vi "Result inspection.vi"(7 "입력 클러스터":T1, 8 "error in":errorcluster caption="에러 입력(에러 없음)", 9 "Ref. Data (excluded)":refnum<vi>[](array[refnum]), 10 "Ref. Data (Inspection)":refnum<vi>[](array[refnum]), 11 "Func ext":string) -> (0 "error out":errorcluster caption="에러 출력", 1 "Data 3D":string[][][][](array[string]), 2 "Data (spec 미적용)":string[][](array[string]), 3 "Data (spec 적용)":string[][](array[string]))   [LabVIEW 2020]
uses:
  Controls/Clst_Result inspec.ctl
  Controls/Cmd_Var Data IO.ctl
  Variables/Global_Cal Info.vi
  Public/Polymorph/Rmv Empt Arr_2D Str.vi
  Public/Polymorph/Cell Space_Table.vi
  Public/Polymorph/Data Class_2D Str.vi
  <vilib>/express/express arith-compare/Formula/XNode/ExpressFormulaBlockNode.xnode
panel:
  out "spec DBL":dbl[][][](array[numeric])
  out "Spec":string[][](array[string])
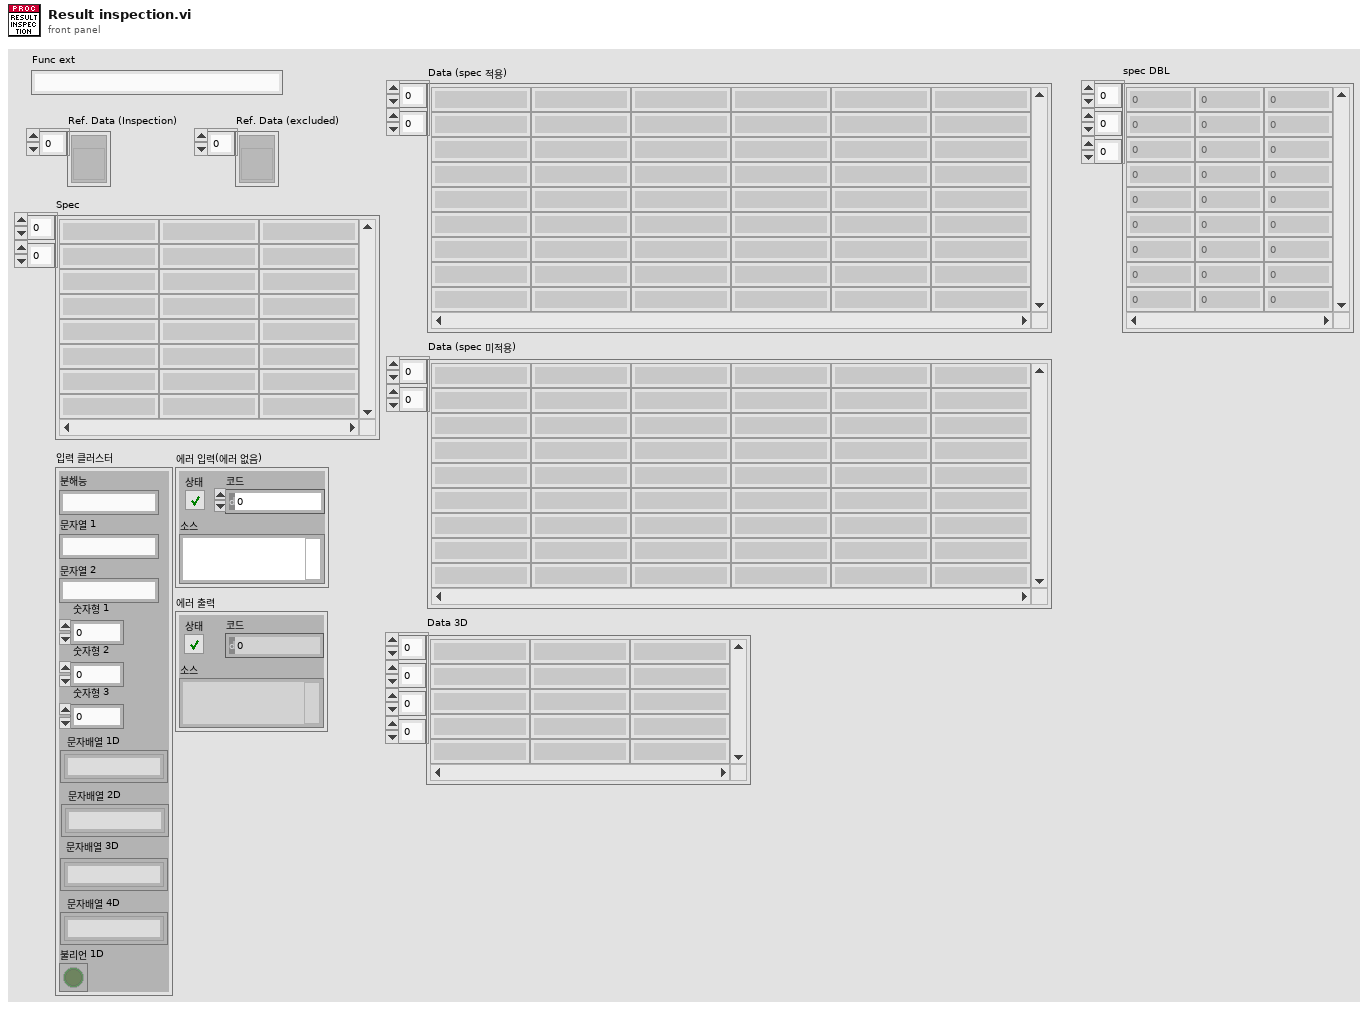
[diagram p1: front panel]
types:
  T1 = typedef "Clst_Result inspec.ctl" = cluster{"분해능":string, "문자열 1":string, "문자열 2":string, "숫자형 1":i32, "숫자형 2":i32, "숫자형 3":dbl, "문자배열 1D":string[], "문자배열 2D":string[][], "문자배열 3D":string[][][], "문자배열 4D":string[][][][], "불리언 1D":bool[]}
  T2 = typedef "Cmd_Var Data IO.ctl" = enum16{"Condition", "Condition Default", "Condition_Temp", "Resolution", "Resolution Default", "Resolution Old", "Spec", "Spec Default", "Spec Old", "Spec Temp", "Result", "Result2", "Result3", "Result_Temp", "Result_ADJ", "Result_ADJ2", "STD1", "STD2", "STD3", "STD4", "STD5", "STD Temp", "CMC", "CMC Default"}
  T3 = cluster{"세부분류코드":string, "형식":string, "옵션":string, "측정기명":string, "EXCEL파일명":string, "TEMP":string}
  T4 = enum8{"Enabled", "Disabled", "Disabled and Grayed Out"}
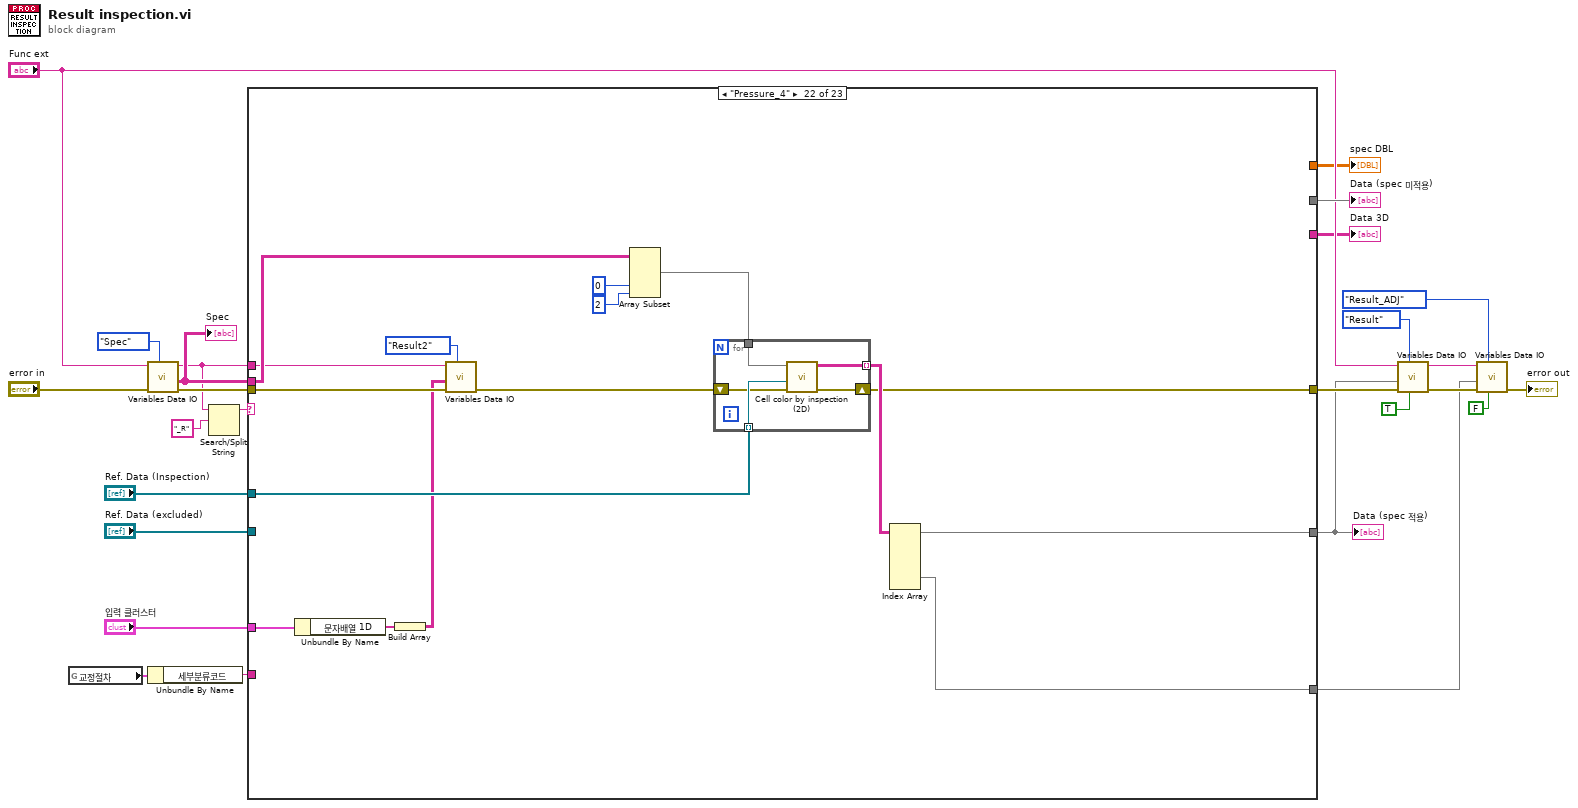
[diagram p0: block diagram]
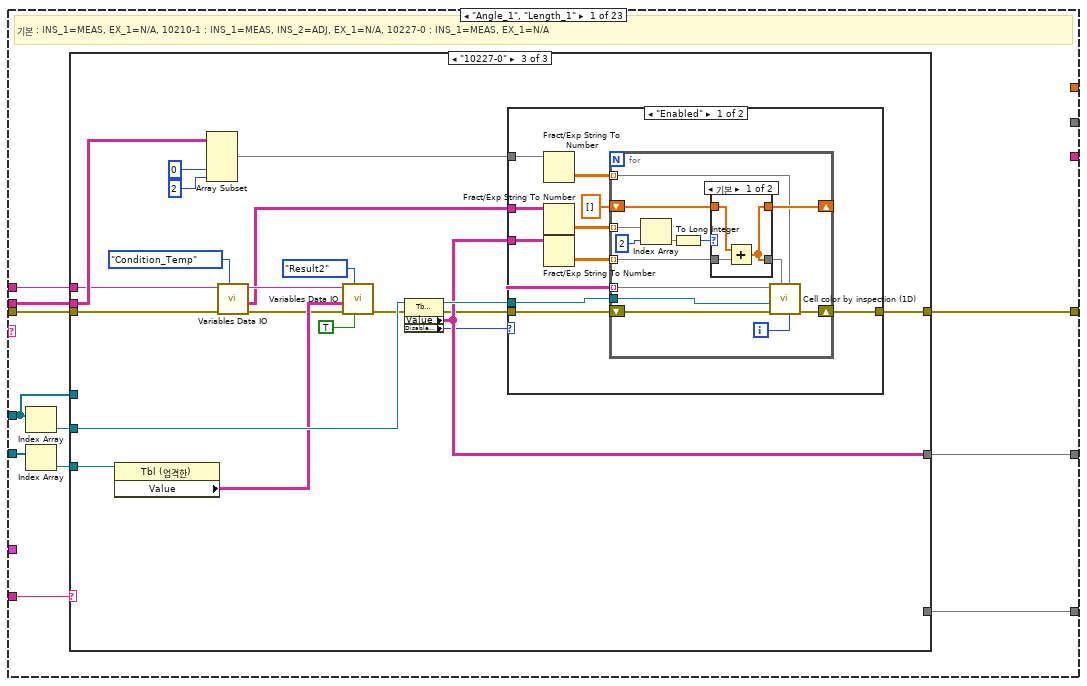
[diagram p2: hidden frame]
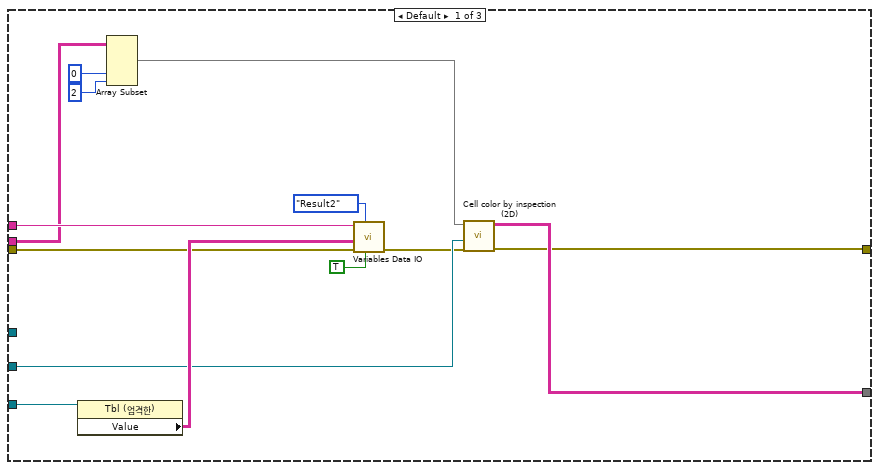
[diagram p3: hidden frame]
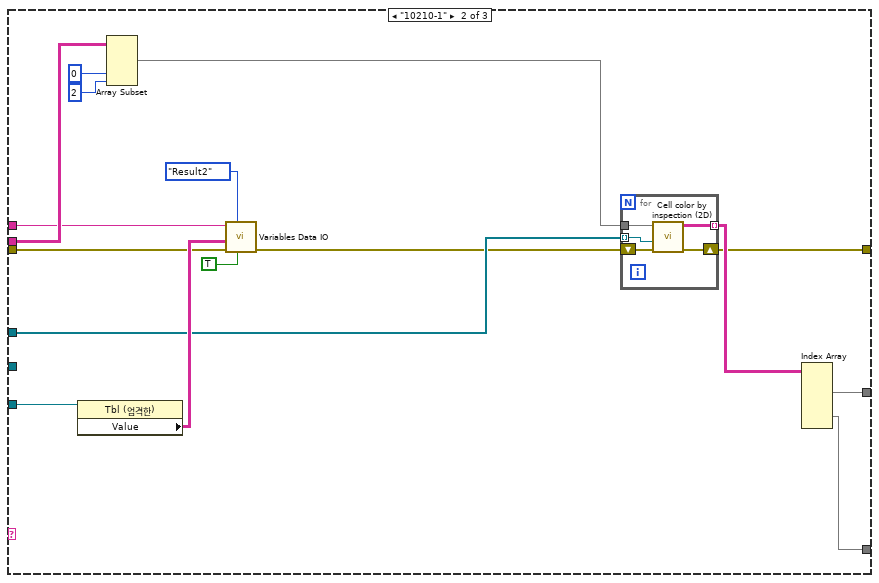
[diagram p4: hidden frame]
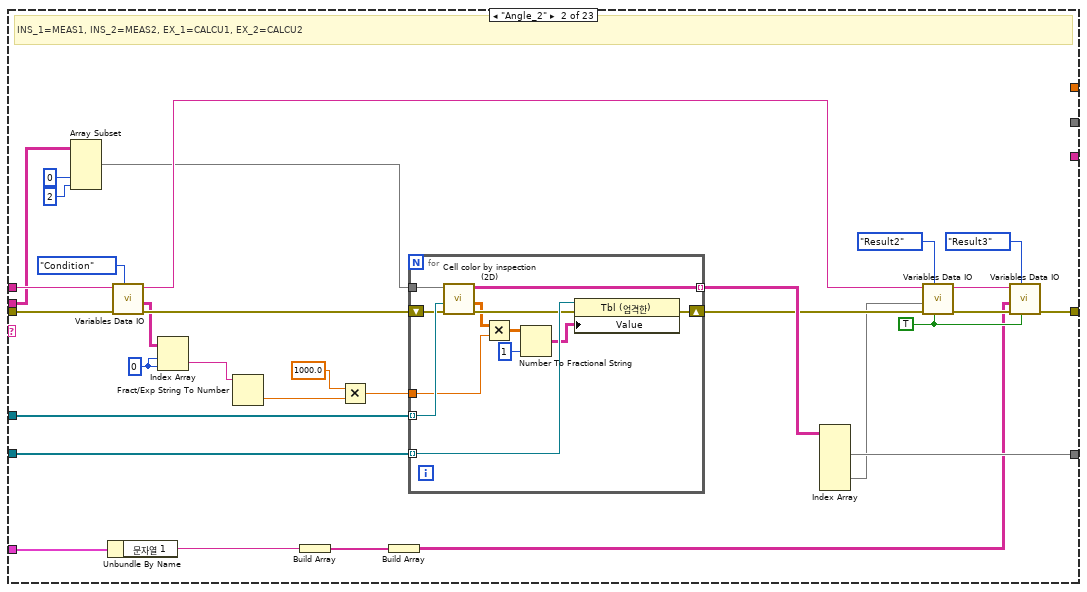
[diagram p7: hidden frame]
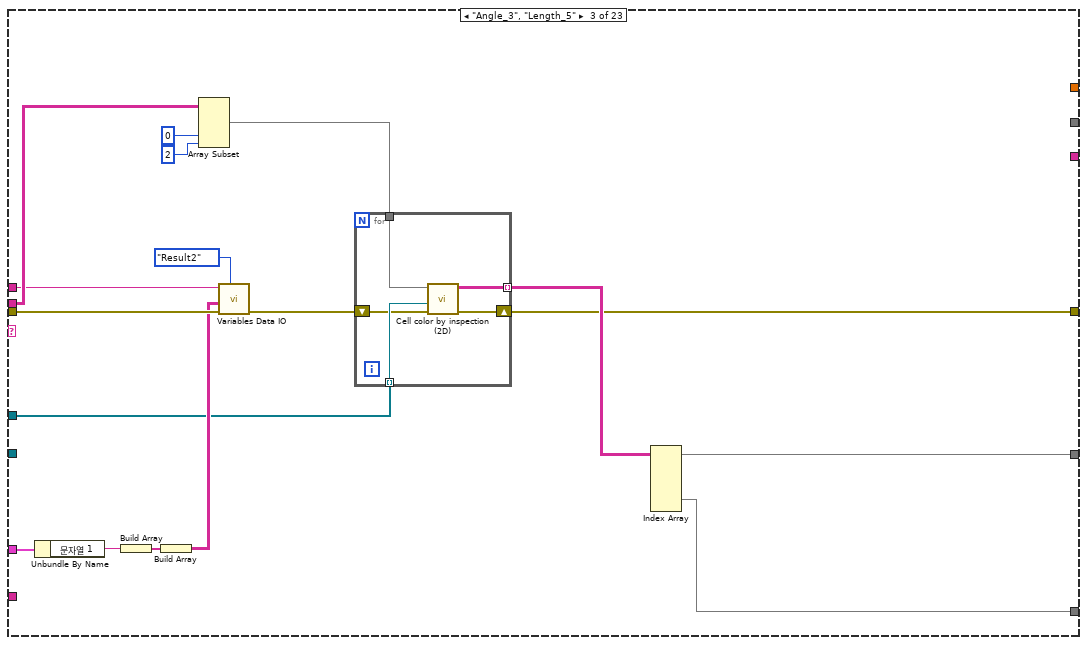
[diagram p8: hidden frame]
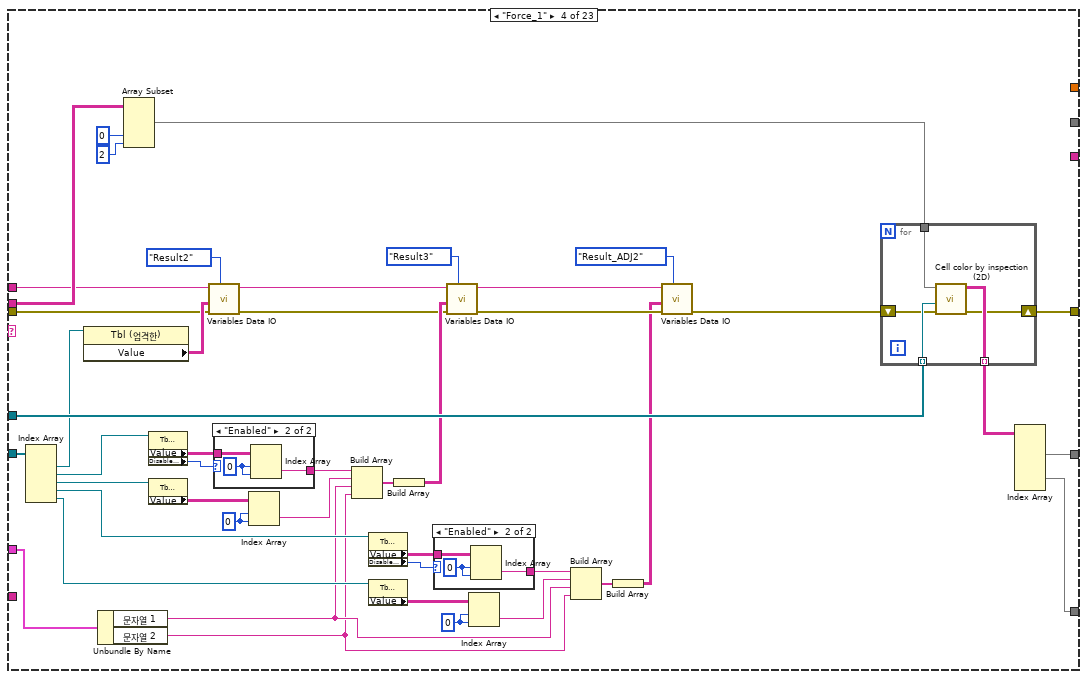
[diagram p9: hidden frame]
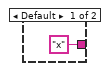
[diagram p10: hidden frame]
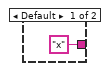
[diagram p11: hidden frame]
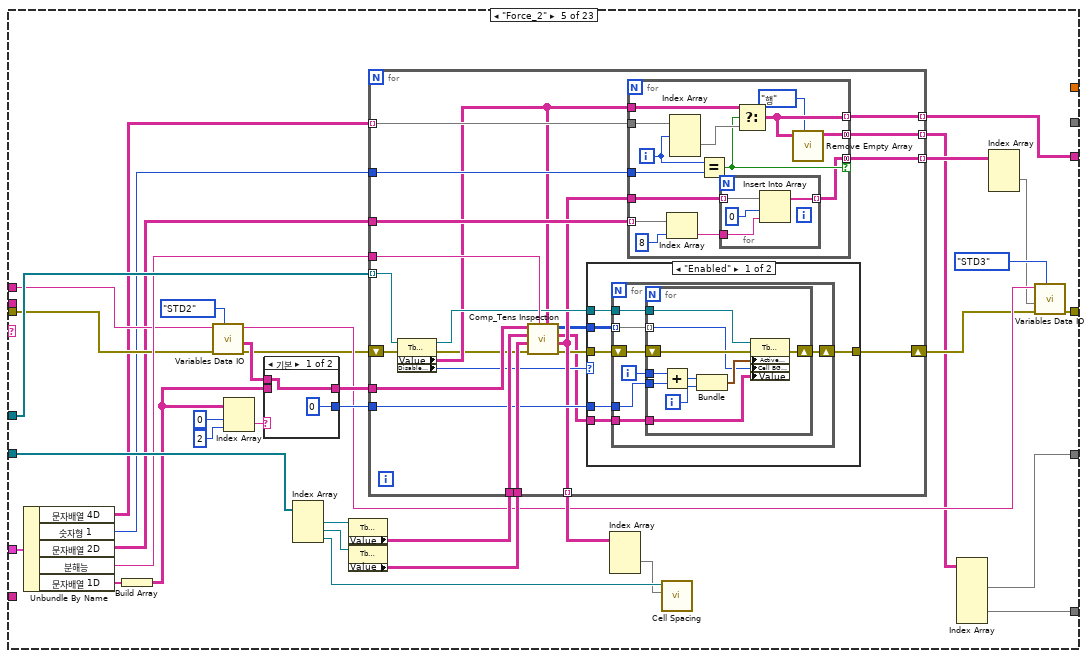
[diagram p12: hidden frame]
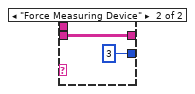
[diagram p14: hidden frame]
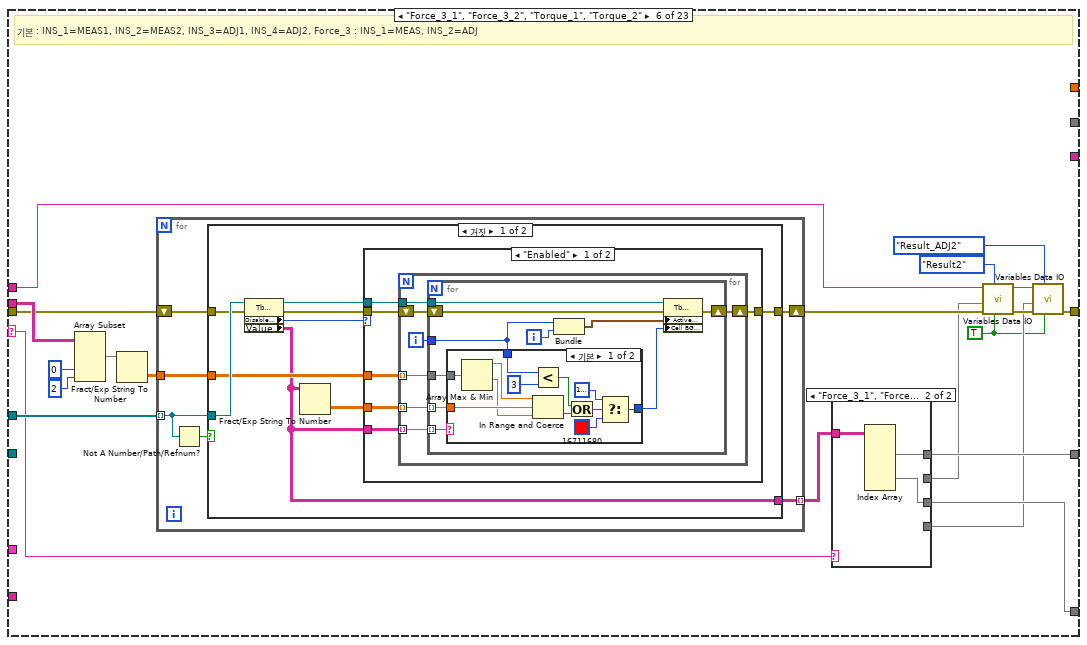
[diagram p15: hidden frame]
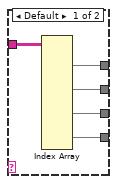
[diagram p16: hidden frame]
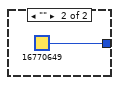
[diagram p17: hidden frame]
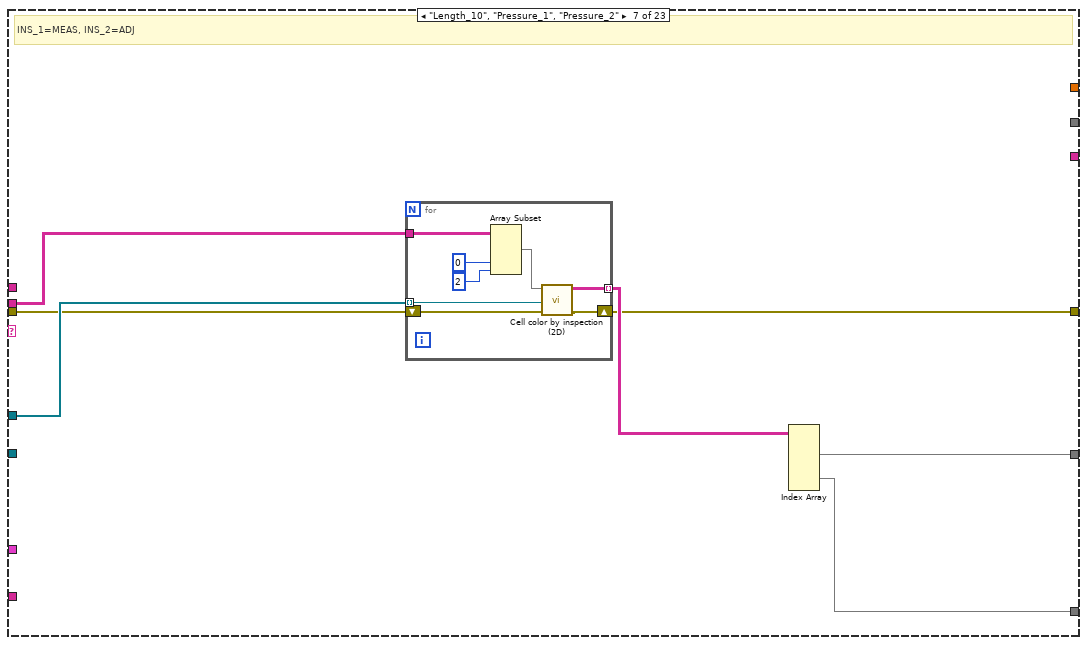
[diagram p20: hidden frame]
diagram:
  n1 = global read "Global_Cal Info.vi" "교정절차"() -> (w10:T3)
  n2 = call "Variables Data IO.vi"("Select"=Cmd_Var_Data_IO."Spec", "error in"="error in", "Func_ext"="Func ext") -> ("error out"=w19:errorcluster, "Data Out"=w17:string[][], "Func_ext Out"=w11:string)  [unwired: 6 in]
  "Spec" <- w17
  n3 = Unbundle By Name(w10) -> ("세부분류코드"=w9:string)
  n4 = Search/Split String(string=w11, search string/char (-)="_R" ("검색 문자열/문자 (-)")) -> (substring before match=w12:string)  [unwired: 1 in, 2 out]
  n5 = case shown="\"Pressure_4\"" w12 {
    selector: w12 -> [_ _ _ _ _ w350 _ _ _ _ _ _ _ _ _ _ _ _ _ _ _ _ _]
    tunnel: w19 -> [w31 w146 w175 w211 w273 w363 w436 w481 w559 w584 w641 w1221 w1258 w1298 w1353 w1411 w1441 w1461 w1514 w1585 w1673 w1691 w1719]
    tunnel: [w30 w131 w168 w206 w253 w356 w433 w448 w536 w579 w622 w1222 w1256 w1294 w1337 w1408 w1443 w1458 w1534 w1615 w1667 w1695 w1709] -> w24
    tunnel: "Ref. Data (Inspection)" -> [w28 w153 w171 w232 w281 w364 w438 w480 w560 w580 w649 w1243 w1260 w1313 w1356 w1415 w1444 w1454 w1542 w1623 w1670 w1697 w1721]
    tunnel: "Ref. Data (excluded)" -> [w34 w147 _ w227 w279 _ _ w483 w551 w577 w648 w1229 w1270 _ w1355 w1410 w1442 w1489 w1505 w1612 _ _ _]
    tunnel: [w36 w151 w167 w205 w247 w360 w434 w475 w534 w578 w610 w1223 w1262 w1310 w1359 w1414 w1439 w1456 w1532 w1613 w1666 w1694 w1717] -> w21
    tunnel: [_ _ _ _ _ _ _ _ _ _ w612 _ _ _ _ _ _ _ w1527 w1606 _ _ _] -> w20
    tunnel: w17 -> [w35 w140 w180 w229 _ w366 w437 w484 w544 w581 w650 w1240 w1265 w1306 w1358 w1413 _ w1469 w1540 w1621 w1678 w1699 w1720]
    tunnel: "입력 클러스터" -> [_ w133 w179 w213 w278 _ _ _ w552 _ w637 w1233 w1272 w1302 _ _ _ w1475 w1516 w1582 w1677 w1692 _]
    tunnel: w11 -> [w32 w145 w177 w212 w272 w351 _ w477 w557 _ w638 w1220 w1276 w1297 w1354 w1409 _ w1462 w1515 w1584 w1675 w1690 w1714]
    tunnel: w9 -> [w29 _ _ _ _ _ _ _ _ _ _ _ _ _ _ w1397 _ _ _ _ _ _ _]
    tunnel: [w27 _ w166 w204 w246 w358 w432 w459 _ _ _ _ w1261 _ _ _ _ w1455 _ _ w1665 w1693 _] -> w4
    tunnel: [_ _ _ _ w257 _ _ _ _ _ _ _ _ _ _ _ _ _ _ _ _ _ _] -> w2
    tunnel: [_ _ _ _ _ _ _ _ _ w576 _ _ _ _ _ _ _ _ _ _ _ _ _] -> w1
    frame "Angle_1", "Length_1" {
      # "기본 : INS_1=MEAS, EX_1=N/A, 10210-1 : INS_1=MEAS, INS_2=ADJ, EX_1=N/A, 10227-0 : INS_1=MEAS, EX_1=N/A"
      n6 = Index Array(array=w28) -> (element=w37:refnum<vi>)  [unwired: 1 in]
      n7 = Index Array(array=w34) -> (element=w33:refnum<vi>)  [unwired: 1 in]
      n8 = case shown="\"10227-0\"" w29 {
        tunnel: w37 -> [w42 _ w93]
        tunnel: [w41 w56 w81] -> w36
        tunnel: w35 -> [w44 w65 w89]
        tunnel: w33 -> [w49 w63 w88]
        tunnel: w32 -> [w47 w61 w84]
        tunnel: w31 -> [w40 w54 w74]
        tunnel: [w38 w52 w78] -> w30
        tunnel: w28 -> [_ w58 _]
        tunnel: [_ w55 _] -> w27
        frame Default {
          n9 = property class="Tbl (엄격한)"(reference=w49) -> ("Value"=w45:string[][])  [unwired: 1 in, 2 out]
          n10 = Array Subset(array=w44, index (col)=0 ("인덱스"), length (col)=2 ("길이")) -> (w43:string[][])  [unwired: 2 in]
          n11 = call "Variables Data IO.vi"("Write blank data ?(F)"=TRUE ("Write blank data ?(T)"), "Select"=Cmd_Var_Data_IO."Result2", "error in"=w40, "Data In"=w45, "Func_ext"=w47) -> ("error out"=w39:errorcluster)  [unwired: 4 in, 2 out]
          n12 = call "Cell color by inspection (2D).vi"("에러 입력(에러 없음)"=w39, "테이블 입력"=w42, "Spec"=w43) -> ("에러 출력"=w38:errorcluster, "Data(str)"=w41:string[][])  [unwired: 6 in, 1 out]
        }
        frame "10210-1" {
          n13 = property class="Tbl (엄격한)"(reference=w63) -> ("Value"=w59:string[][])  [unwired: 1 in, 2 out]
          n14 = Array Subset(array=w65, index (col)=0 ("인덱스"), length (col)=2 ("길이")) -> (w64:string[][])  [unwired: 2 in]
          n15 = call "Variables Data IO.vi"("Write blank data ?(F)"=TRUE ("Write blank data ?(T)"), "Select"=Cmd_Var_Data_IO."Result2", "error in"=w54, "Data In"=w59, "Func_ext"=w61) -> ("error out"=w53:errorcluster)  [unwired: 4 in, 2 out]
          n16 = for {
            tunnel: [w69] -> w57 mode=indexing
            tunnel: w64 -> [w72]
            tunnel: w58 -> [w70] mode=indexing
            shift-right: [w68] -> w52
            shift-left: w53 -> [w71]
            n17 = call "Cell color by inspection (2D).vi"("에러 입력(에러 없음)"=w71, "테이블 입력"=w70, "Spec"=w72) -> ("에러 출력"=w68:errorcluster, "Data(str)"=w69:string[][])  [unwired: 6 in, 1 out]
          }
          n18 = Index Array(array=w57) -> (element #1=w56:string[][], element #2=w55:string[][])  [unwired: 6 in]
        }
        frame "10227-0" {
          n19 = property class="Tbl (엄격한)"(reference=w88) -> ("Value"=w85:string[][])  [unwired: 1 in, 2 out]
          n20 = Array Subset(array=w89, index (col)=0 ("인덱스"), length (col)=2 ("길이")) -> (w79:string[][])  [unwired: 2 in]
          n21 = call "Variables Data IO.vi"("Select"=Cmd_Var_Data_IO."Condition_Temp", "error in"=w74, "Func_ext"=w84) -> ("error out"=w75:errorcluster, "Data Out"=w80:string[][], "Func_ext Out"=w83:string)  [unwired: 6 in]
          n22 = call "Variables Data IO.vi"("Write blank data ?(F)"=TRUE ("Write blank data ?(T)"), "Select"=Cmd_Var_Data_IO."Result2", "error in"=w75, "Data In"=w85, "Func_ext"=w83) -> ("error out"=w76:errorcluster)  [unwired: 4 in, 2 out]
          n23 = property class="Tbl (엄격한)"(reference=w93, error in=w76) -> (reference out=w92:refnum<vi>, error out=w77:errorcluster, "Value"=w81:string[][], "DisabledEnum"=w73:T4)
          n24 = case shown="\"Enabled\"" w73 {
            tunnel: w92 -> [w102 _]
            tunnel: w81 -> [w101 _]
            tunnel: w80 -> [w100 _]
            tunnel: w79 -> [w99 _]
            tunnel: [w95 w123] -> w78
            tunnel: w77 -> [w94 w123]
            frame "Enabled" {
              n25 = Fract/Exp String To Number(string=w99) -> (number=w103:dbl[][])  [unwired: 3 in, 1 out]
              n26 = Fract/Exp String To Number(string=w100) -> (number=w96:dbl[][])  [unwired: 3 in, 1 out]
              n27 = Fract/Exp String To Number(string=w101) -> (number=w98:dbl[][])  [unwired: 3 in, 1 out]
              n28 = for {
                tunnel: w103 -> [w110] mode=indexing
                tunnel: w98 -> [w116] mode=indexing
                tunnel: w102 -> [w107]
                tunnel: w101 -> [w106] mode=indexing
                shift-right: [w105] -> w95
                shift-left: w94 -> [w108]
                shift-right: [w111] -> _
                shift-left: dbl[] [] -> [w117]
                tunnel: w96 -> [w113] mode=indexing
                i -> [w104]
                n29 = Index Array(array=w113, index=2 ("인덱스")) -> (element=w115:dbl)
                n30 = To Long Integer(number=w115) -> (32bit integer=w112:i32)
                n31 = case shown="기본" w112 {
                  tunnel: w116 -> [w119 w122]
                  tunnel: [w118 w122] -> w109
                  tunnel: w117 -> [w120 w121]
                  tunnel: [w118 w121] -> w111
                  frame Default {
                    n32 = Add(x=w120, y=w119) -> (x+y=w118:dbl[])
                  }
                  frame 0 {
                  }
                }
                n33 = call "Cell color by inspection (1D).vi"("행번호"=w104, "Spec"=w110, "Data (DBL)"=w109, "에러 입력"=w108, "테이블 입력"=w107, "Data (str)"=w106) -> ("에러 출력"=w105:errorcluster)  [unwired: 5 in]
              }
            }
            frame Default {
            }
          }
        }
      }
    }
    frame "Angle_2" {
      w138 = 0 ("인덱스 (열)")
      w130 = TRUE ("Write blank data ?")
      # "INS_1=MEAS1, INS_2=MEAS2, EX_1=CALCU1, EX_2=CALCU2"
      n34 = Array Subset(array=w140, index (col)=0 ("인덱스"), length (col)=2 ("길이")) -> (w124:string[][])  [unwired: 2 in]
      n35 = Unbundle By Name(w133) -> ("문자열 1"=w127:string)
      n36 = call "Variables Data IO.vi"("Select"=Cmd_Var_Data_IO."Condition", "error in"=w146, "Func_ext"=w145) -> ("Data Out"=w142:string[][], "Func_ext Out"=w144:string)  [unwired: 6 in, 1 out]
      n37 = Index Array(array=w142, index (row)=w138, index (col)=w138) -> (element=w137:string)
      n38 = Fract/Exp String To Number(string=w137) -> (number=w136:dbl)  [unwired: 3 in, 1 out]
      n39 = Build Array(w127) -> (w126:string[])
      n40 = Multiply(x=1000.0 ("y"), y=w136) -> (x*y=w135:dbl)
      n41 = Build Array(w126) -> (w125:string[][])
      n42 = for {
        tunnel: w153 -> [w165] mode=indexing
        tunnel: [w159] -> w152 mode=indexing
        shift-right: [w160] -> w149
        shift-left: w146 -> [w164]
        tunnel: w147 -> [w162] mode=indexing
        tunnel: w124 -> [w163]
        tunnel: w135 -> [w157]
        n43 = call "Cell color by inspection (2D).vi"("에러 입력(에러 없음)"=w164, "테이블 입력"=w165, "Spec"=w163) -> ("에러 출력"=w161:errorcluster, "Data(DBL)"=w158:dbl[][], "Data(str)"=w159:string[][])  [unwired: 6 in]
        n44 = Multiply(x=w158, y=w157) -> (x*y=w156:dbl[][])
        n45 = Number To Fractional String(number=w156, precision (6)=i16 1 ("정밀도(6)")) -> (F-format string=w154:string[][])  [unwired: 2 in]
        n46 = property class="Tbl (엄격한)"(reference=w162, error in=w161, "Value"=w154) -> (error out=w160:errorcluster)  [unwired: 1 out]
      }
      n47 = Index Array(array=w152) -> (element #1=w151:string[][], element #2=w148:string[][])  [unwired: 6 in]
      n48 = call "Variables Data IO.vi"("Write blank data ?(F)"=w130, "Select"=Cmd_Var_Data_IO."Result2", "error in"=w149, "Data In"=w148, "Func_ext"=w144) -> ("error out"=w132:errorcluster, "Func_ext Out"=w128:string)  [unwired: 4 in, 1 out]
      n49 = call "Variables Data IO.vi"("Write blank data ?(F)"=w130, "Select"=Cmd_Var_Data_IO."Result3", "error in"=w132, "Data In"=w125, "Func_ext"=w128) -> ("error out"=w131:errorcluster)  [unwired: 4 in, 2 out]
    }
    frame "Angle_3", "Length_5" {
      n50 = Unbundle By Name(w179) -> ("문자열 1"=w176:string)
      n51 = Build Array(w176) -> (w174:string[])
      n52 = Build Array(w174) -> (w173:string[][])
      n53 = Array Subset(array=w180, index (col)=0 ("인덱스"), length (col)=2 ("길이")) -> (w172:string[][])  [unwired: 2 in]
      n54 = call "Variables Data IO.vi"("Select"=Cmd_Var_Data_IO."Result2", "error in"=w175, "Data In"=w173, "Func_ext"=w177) -> ("error out"=w170:errorcluster)  [unwired: 5 in, 2 out]
      n55 = for {
        tunnel: w172 -> [w187]
        tunnel: w171 -> [w186] mode=indexing
        tunnel: [w184] -> w169 mode=indexing
        shift-right: [w183] -> w168
        shift-left: w170 -> [w185]
        n56 = call "Cell color by inspection (2D).vi"("에러 입력(에러 없음)"=w185, "테이블 입력"=w186, "Spec"=w187) -> ("에러 출력"=w183:errorcluster, "Data(str)"=w184:string[][])  [unwired: 6 in, 1 out]
      }
      n57 = Index Array(array=w169) -> (element #1=w167:string[][], element #2=w166:string[][])  [unwired: 6 in]
    }
    frame "Force_1" {
      w196 = 0 ("인덱스 (행)")
      w218 = 0 ("인덱스 (행)")
      n58 = Index Array(array=w227) -> (element #1=w226:refnum<vi>, element #2=w224:refnum<vi>, element #3=w223:refnum<vi>, element #4=w192:refnum<vi>, element #5=w191:refnum<vi>)  [unwired: 5 in]
      n59 = property class="Tbl (엄격한)"(reference=w226) -> ("Value"=w225:string[][])  [unwired: 1 in, 2 out]
      n60 = Unbundle By Name(w213) -> ("문자열 1"=w189:string, "문자열 2"=w188:string)
      n61 = Array Subset(array=w229, index (col)=0 ("인덱스"), length (col)=2 ("길이")) -> (w209:string[][])  [unwired: 2 in]
      n62 = property class="Tbl (엄격한)"(reference=w224) -> ("Value"=w220:string[][], "DisabledEnum"=w221:T4)  [unwired: 1 in, 2 out]
      n63 = property class="Tbl (엄격한)"(reference=w223) -> ("Value"=w217:string[][])  [unwired: 1 in, 2 out]
      n64 = call "Variables Data IO.vi"("Select"=Cmd_Var_Data_IO."Result2", "error in"=w211, "Data In"=w225, "Func_ext"=w212) -> ("error out"=w207:errorcluster, "Func_ext Out"=w210:string)  [unwired: 5 in, 1 out]
      n65 = case shown="\"Enabled\"" w221 {
        tunnel: w220 -> [_ w245]
        tunnel: ["ⅹ" w243] -> w219
        frame Default {
        }
        frame "Enabled" {
          w244 = 0 ("인덱스 (행)")
          n66 = Index Array(array=w245, index (row)=w244, index (col)=w244) -> (element=w243:string)
        }
      }
      n67 = Index Array(array=w217, index (row)=w218, index (col)=w218) -> (element=w216:string)
      n68 = Build Array(w219, w216, w189, w188) -> (w215:string[])
      n69 = property class="Tbl (엄격한)"(reference=w192) -> ("Value"=w194:string[][], "DisabledEnum"=w193:T4)  [unwired: 1 in, 2 out]
      n70 = property class="Tbl (엄격한)"(reference=w191) -> ("Value"=w197:string[][])  [unwired: 1 in, 2 out]
      n71 = Build Array(w215) -> (w214:string[][])
      n72 = case shown="\"Enabled\"" w193 {
        tunnel: w194 -> [_ w236]
        tunnel: ["ⅹ" w234] -> w195
        frame Default {
        }
        frame "Enabled" {
          w235 = 0 ("인덱스 (행)")
          n73 = Index Array(array=w236, index (row)=w235, index (col)=w235) -> (element=w234:string)
        }
      }
      n74 = call "Variables Data IO.vi"("Select"=Cmd_Var_Data_IO."Result3", "error in"=w207, "Data In"=w214, "Func_ext"=w210) -> ("error out"=w202:errorcluster, "Func_ext Out"=w200:string)  [unwired: 5 in, 1 out]
      n75 = Index Array(array=w197, index (row)=w196, index (col)=w196) -> (element=w198:string)
      n76 = Build Array(w195, w198, w189, w188) -> (w199:string[])
      n77 = Build Array(w199) -> (w190:string[][])
      n78 = call "Variables Data IO.vi"("Select"=Cmd_Var_Data_IO."Result_ADJ2", "error in"=w202, "Data In"=w190, "Func_ext"=w200) -> ("error out"=w201:errorcluster)  [unwired: 5 in, 2 out]
      n79 = for {
        tunnel: w209 -> [w241]
        tunnel: w232 -> [w240] mode=indexing
        tunnel: [w239] -> w208 mode=indexing
        shift-right: [w237] -> w206
        shift-left: w201 -> [w238]
        n80 = call "Cell color by inspection (2D).vi"("에러 입력(에러 없음)"=w238, "테이블 입력"=w240, "Spec"=w241) -> ("에러 출력"=w237:errorcluster, "Data(str)"=w239:string[][])  [unwired: 6 in, 1 out]
      }
      n81 = Index Array(array=w208) -> (element #1=w205:string[][], element #2=w204:string[][])  [unwired: 6 in]
    }
    frame "Force_2" {
      n82 = Unbundle By Name(w278) -> ("문자배열 4D"=w260:string[][][][], "숫자형 1"=w261:i32, "문자배열 2D"=w262:string[][], "분해능"=w274:string, "문자배열 1D"=w267:string[])
      n83 = Build Array(w267) -> (w263:string[][])
      n84 = call "Variables Data IO.vi"("Select"=Cmd_Var_Data_IO."STD2", "error in"=w273, "Func_ext"=w272) -> ("error out"=w252:errorcluster, "Data Out"=w265:string[][], "Func_ext Out"=w254:string)  [unwired: 6 in]
      n85 = Index Array(array=w263, index (row)=0 ("비활성화된 인덱스 (행)"), index (col)=2 ("비활성화된 인덱스 (열)")) -> (element=w268:string)
      n86 = case shown="기본" w268 {
        tunnel: w263 -> [_ w349]
        tunnel: [w347 w349] -> w266
        tunnel: w265 -> [w347 _]
        tunnel: [0 ("x") 3 ("x")] -> w264
        frame Default {
        }
        frame "Force Measuring Device" {
        }
      }
      n87 = Index Array(array=w279) -> (element #1=w280:refnum<vi>, element #2=w277:refnum<vi>, element #3=w259:refnum<vi>)  [unwired: 3 in]
      n88 = property class="Tbl (엄격한)"(reference=w280) -> ("Value"=w276:string[][])  [unwired: 1 in, 2 out]
      n89 = property class="Tbl (엄격한)"(reference=w277) -> ("Value"=w275:string[][])  [unwired: 1 in, 2 out]
      n90 = for {
        tunnel: w276 -> [w303]
        tunnel: w275 -> [w302]
        tunnel: w274 -> [w301]
        tunnel: w266 -> [w300]
        tunnel: w264 -> [w299]
        tunnel: w262 -> [w298]
        tunnel: w261 -> [w297]
        tunnel: w260 -> [w296] mode=indexing
        tunnel: [w293] -> w258 mode=indexing
        tunnel: [w292] -> w257 mode=indexing
        tunnel: w281 -> [w291] mode=indexing
        tunnel: [w290] -> w255 mode=indexing
        shift-right: [w287] -> w251
        shift-left: w252 -> [w289]
        tunnel: [w286] -> w248 mode=indexing
        n91 = property class="Tbl (엄격한)"(reference=w291, error in=w289) -> (reference out=w295:refnum<vi>, error out=w288:errorcluster, "Value"=w294:string[][], "DisabledEnum"=w285:T4)
        n92 = call "Comp_Tens Inspection.vi"("Value"=w294, "분해능"=w301, "error in (no error)"=w288, "Spec"=w302, "Condition"=w303, "STD"=w300) -> ("error out"=w283:errorcluster, "사용기준추"=w293:string[][], "Value out"=w282:string[][], "색상 배열"=w284:u32[][])  [unwired: 2 in]
        n93 = case shown="\"Enabled\"" w285 {
          tunnel: w299 -> [w309 _]
          tunnel: w295 -> [w308 _]
          tunnel: [w307 w327] -> w287
          tunnel: w284 -> [w306 _]
          tunnel: w283 -> [w305 w327]
          tunnel: w282 -> [w304 _]
          frame "Enabled" {
            n94 = for {
              tunnel: w306 -> [w316] mode=indexing
              tunnel: w308 -> [w315]
              shift-right: [w312] -> w307
              shift-left: w305 -> [w313]
              tunnel: w304 -> [w311]
              tunnel: w309 -> [w310]
              i -> [w314]
              n95 = for {
                tunnel: w316 -> [w319] mode=indexing
                tunnel: w315 -> [w326]
                tunnel: w314 -> [w321]
                shift-right: [w322] -> w312
                shift-left: w313 -> [w323]
                tunnel: w311 -> [w318]
                tunnel: w310 -> [w317]
                i -> [w325]
                n96 = Add(x=w321, y=w317) -> (x+y=w320:i32)
                n97 = Bundle(w320, w325) -> (w324:cluster{i32, i32})  [unwired: 1 in]
                n98 = property class="Tbl (엄격한)"(reference=w326, error in=w323, "Active Cell"=w324, "Cell BG Color"=w319, "Value"=w318) -> (error out=w322:errorcluster)  [unwired: 1 out]
              }
            }
          }
          frame Default {
          }
        }
        n99 = for {
          tunnel: w296 -> [w340]
          tunnel: w294 -> [w337]
          tunnel: w297 -> [w341]
          tunnel: [w336] -> w292 mode=indexing
          tunnel: w298 -> [w330] mode=indexing
          tunnel: [w335] -> w286 mode=concatenating
          tunnel: w293 -> [w332]
          tunnel: [w331] -> w290 mode=concatenating if=w333
          i -> [w339]
          n100 = Index Array(array=w330, index=8 ("비활성화된 인덱스 (열)")) -> (element=w328:string)
          n101 = Index Array(array=w340, index (dim 0)=w339) -> (element=w338:string[][])  [unwired: 2 in]
          n102 = Equal?(x=w339, y=w341) -> (x = y?=w333:bool)
          n103 = for {
            tunnel: w332 -> [w345] mode=indexing
            tunnel: w328 -> [w344]
            tunnel: [w342] -> w331 mode=indexing
            n104 = Insert Into Array(array=w345, index=0 ("인덱스"), new element=w344) -> (w342:string[])
          }
          n105 = Select(t=w337, s=w333, f=w338) -> (s? t:f=w336:string[][])
          n106 = call-poly "Remove Empty Array.vi"("조건"=enum16{"행", "열", "행,열"}."행", "Data in"=w336) -> ("Data out"=w335:string[][])  [unwired: 8 in, 1 out]
        }
      }
      n107 = Index Array(array=w258) -> (element=w249:string[][])  [unwired: 3 in]
      n108 = call-poly "Cell Spacing.vi"("Data in"=w249, "테이블 참조 in"=w259) -> ()  [unwired: 7 in, 3 out]
      n109 = Index Array(array=w248) -> (element #1=w247:string[][], element #2=w246:string[][])  [unwired: 6 in]
      n110 = Index Array(array=w255) -> (element=w250:string[][])  [unwired: 3 in]
      n111 = call "Variables Data IO.vi"("Select"=Cmd_Var_Data_IO."STD3", "error in"=w251, "Data In"=w250, "Func_ext"=w254) -> ("error out"=w253:errorcluster)  [unwired: 5 in, 2 out]
    }
    frame "Force_3_1", "Force_3_2", "Torque_1", "Torque_2" {
      w352 = TRUE ("Clear data ?")
      # "기본 : INS_1=MEAS1, INS_2=MEAS2, INS_3=ADJ1, INS_4=ADJ2, Force_3 : INS_1=MEAS, INS_2=ADJ"
      n112 = Array Subset(array=w366, index (col)=0 ("인덱스"), length (col)=2 ("길이")) -> (w369:string[][])  [unwired: 2 in]
      n113 = Fract/Exp String To Number(string=w369) -> (number=w365:dbl[][])  [unwired: 3 in, 1 out]
      n114 = for {
        tunnel: w364 -> [w384] mode=indexing
        tunnel: w365 -> [w382]
        tunnel: [w381] -> w361 mode=indexing
        shift-right: [w379] -> w362
        shift-left: w363 -> [w380]
        n115 = Not A Number/Path/Refnum?(number/path/refnum=w384) -> (NaN/Path/Refnum?=w383:bool)
        n116 = case shown="거짓" w383 {
          tunnel: w382 -> [w391 _]
          tunnel: [w390 _] -> w381
          tunnel: w384 -> [w393 _]
          tunnel: w380 -> [w388 w431]
          tunnel: [w386 w431] -> w379
          frame False {
            n117 = property class="Tbl (엄격한)"(reference=w393, error in=w388) -> (reference out=w392:refnum<vi>, error out=w387:errorcluster, "DisabledEnum"=w385:T4, "Value"=w390:string[][])
            n118 = Fract/Exp String To Number(string=w390) -> (number=w389:dbl[][])  [unwired: 3 in, 1 out]
            n119 = case shown="\"Enabled\"" w385 {
              tunnel: w392 -> [w399 _]
              tunnel: w391 -> [w398 _]
              tunnel: w390 -> [w397 _]
              tunnel: w389 -> [w396 _]
              tunnel: w387 -> [w395 w430]
              tunnel: [w394 w430] -> w386
              frame "Enabled" {
                n120 = for {
                  tunnel: w398 -> [w402] mode=indexing
                  tunnel: w396 -> [w406] mode=indexing
                  tunnel: w399 -> [w405]
                  tunnel: w397 -> [w404] mode=indexing
                  shift-right: [w400] -> w394
                  shift-left: w395 -> [w401]
                  i -> [w403]
                  n121 = for {
                    tunnel: w402 -> [w411]
                    tunnel: w406 -> [w412] mode=indexing
                    tunnel: w405 -> [w416]
                    tunnel: w404 -> [w410] mode=indexing
                    tunnel: w403 -> [w409]
                    shift-right: [w407] -> w400
                    shift-left: w401 -> [w408]
                    i -> [w415]
                    n122 = case shown="기본" w410 {
                      tunnel: w412 -> [w428 _]
                      tunnel: [w426 u32 16770649] -> w413
                      tunnel: w411 -> [w424 _]
                      tunnel: w409 -> [w417 _]
                      frame Default {
                        n123 = Array Max & Min(array=w424) -> (max value=w423:dbl, min value=w422:dbl)  [unwired: 2 out]
                        n124 = Less?(x=w417, y=3) -> (x < y?=w419:bool)
                        n125 = In Range and Coerce(upper limit=w423, x=w428, lower limit=w422) -> (In Range?=w420:bool)  [unwired: 1 out]
                        n126 = Or(x=w419, y=w420) -> (x .or. y?=w418:bool)
                        n127 = Select(t=u32 16777226, s=w418, f=u32 16711680) -> (s? t:f=w426:u32)
                      }
                      frame "" {
                      }
                    }
                    n128 = Bundle(w409, w415) -> (w414:cluster{i32, i32})  [unwired: 1 in]
                    n129 = property class="Tbl (엄격한)"(reference=w416, error in=w408, "Active Cell"=w414, "Cell BG Color"=w413) -> (error out=w407:errorcluster)  [unwired: 1 out]
                  }
                }
              }
              frame Default {
              }
            }
          }
          frame True {
          }
        }
      }
      n130 = case shown="\"Force_3_1\", \"Force_3_2\"" w350 {
        tunnel: w361 -> [w375 w378]
        tunnel: [w374 w377] -> w360
        tunnel: [w373 _] -> w359
        tunnel: [w372 w376] -> w358
        tunnel: [w371 _] -> w353
        frame Default {
          n131 = Index Array(array=w375) -> (element #1=w374:string[][], element #2=w373:string[][], element #3=w372:string[][], element #4=w371:string[][])  [unwired: 12 in]
        }
        frame "Force_3_1", "Force_3_2" {
          n132 = Index Array(array=w378) -> (element #1=w377:string[][], element #2=w376:string[][])  [unwired: 6 in]
        }
      }
      n133 = call "Variables Data IO.vi"("Write blank data ?(F)"=w352, "Select"=Cmd_Var_Data_IO."Result2", "error in"=w362, "Data In"=w359, "Func_ext"=w351) -> ("error out"=w357:errorcluster, "Func_ext Out"=w355:string)  [unwired: 4 in, 1 out]
      n134 = call "Variables Data IO.vi"("Write blank data ?(F)"=w352, "Select"=Cmd_Var_Data_IO."Result_ADJ2", "error in"=w357, "Data In"=w353, "Func_ext"=w355) -> ("error out"=w356:errorcluster)  [unwired: 4 in, 2 out]
    }
    frame "Length_10", "Pressure_1", "Pressure_2" {
      # "INS_1=MEAS, INS_2=ADJ"
      n135 = for {
        tunnel: w438 -> [w442] mode=indexing
        tunnel: [w441] -> w435 mode=indexing
        tunnel: w437 -> [w444]
        shift-right: [w439] -> w433
        shift-left: w436 -> [w440]
        n136 = Array Subset(array=w444, index (col)=0 ("인덱스"), length (col)=2 ("길이")) -> (w443:string[][])  [unwired: 2 in]
        n137 = call "Cell color by inspection (2D).vi"("에러 입력(에러 없음)"=w440, "테이블 입력"=w442, "Spec"=w443) -> ("에러 출력"=w439:errorcluster, "Data(str)"=w441:string[][])  [unwired: 6 in, 1 out]
      }
      n138 = Index Array(array=w435) -> (element #1=w434:string[][], element #2=w432:string[][])  [unwired: 6 in]
    }
    frame "Length_12" {
      w447 = TRUE ("Write blank data ?(T)")
      n139 = Index Array(array=w483) -> (element #1=w471:refnum<vi>, element #2=w470:refnum<vi>, element #3=w469:refnum<vi>, element #4=w455:refnum<vi>, element #5=w454:refnum<vi>)  [unwired: 5 in]
      n140 = Array Subset(array=w484, index (col)=0 ("인덱스"), length (col)=2 ("길이")) -> (w461:string[][])  [unwired: 2 in]
      n141 = Build Array(w455, w454) -> (w453:refnum<vi>[])
      n142 = property class="Tbl (엄격한)"(reference=w469) -> ("Row Headers[]"=w452:string[], "Value"=w473:string[][])  [unwired: 1 in, 2 out]
      n143 = for {
        tunnel: [w493] -> w476 mode=indexing
        tunnel: w461 -> [w497]
        tunnel: w480 -> [w496] mode=indexing
        shift-right: [w492] -> w478
        shift-left: w481 -> [w495]
        tunnel: w471 -> [w505]
        tunnel: w470 -> [w503]
        tunnel: w452 -> [w500]
        tunnel: [w499] -> w451
        tunnel: [w498] -> w450 mode=indexing
        n144 = property class="Tbl (엄격한)"(reference=w505) -> ("Value"=w504:string[][])  [unwired: 1 in, 2 out]
        n145 = property class="Tbl (엄격한)"(reference=w503) -> ("Value"=w502:string[][])  [unwired: 1 in, 2 out]
        n146 = call "Cell color by inspection (2D).vi"("에러 입력(에러 없음)"=w495, "테이블 입력"=w496, "Spec"=w497) -> ("에러 출력"=w492:errorcluster, "Data(DBL)"=w494:dbl[][], "Data(str)"=w493:string[][])  [unwired: 6 in]
        n147 = for {
          tunnel: w504 -> [w530] mode=indexing
          tunnel: [w528] -> w501 mode=indexing
          tunnel: w502 -> [w527] mode=indexing
          tunnel: w494 -> [w520] mode=indexing
          n148 = Index Array(array=w530) -> (element #1=w523:string, element #2=w522:string)  [unwired: 2 in]
          n149 = call "Standard Deviation.vi"("X"=w520) -> ("standard deviation"=w521:dbl)  [unwired: 8 in, 2 out]
          n150 = Format Into String(format string="%s_%s" ("포맷 문자열"), w523, w522) -> (resulting string=w529:string)  [unwired: 2 in, 1 out]
          n151 = Index Array(array=w527, index=2 ("인덱스")) -> (element=w525:string)
          n152 = Number To Fractional String(number=w521) -> (F-format string=w524:string)  [unwired: 3 in]
          n153 = Build Array(w529, w523, w522, w525, w524) -> (w528:string[])
        }
        n154 = for {
          tunnel: w501 -> [w519]
          tunnel: w500 -> [w518] mode=indexing
          tunnel: [w516] -> w498 mode=indexing
          tunnel: [w511] -> w499 mode=indexing
          w513 = 0 ("비활성화된 인덱스 (열)")
          n155 = call-poly "Data Classification.vi"("DATA 입력"=w519, "검색 문자열"=w518) -> ("DATA 출력"=w517:string[][])  [unwired: 5 in, 4 out]
          n156 = Index Array(array=w517, index (row) #1=w513, index (col) #1=w513, index (col) #5=4 ("인덱스 (열)")) -> (element #1=w512:string, element #2=w510:string, element #3=w509:string, element #4=w506:string, element #5=w507:string[])  [unwired: 7 in]
          n157 = Fract/Exp String To Number(string=w507) -> (number=w515:dbl[])  [unwired: 3 in, 1 out]
          n158 = Build Array(w512, w510, w509, w506) -> (w511:string[])
          n159 = Array Max & Min(array=w515) -> (max value=w514:dbl)  [unwired: 3 out]
          n160 = Number To Fractional String(number=w514) -> (F-format string=w516:string)  [unwired: 3 in]
        }
      }
      n161 = for {
        tunnel: [w488] -> w460 mode=indexing
        tunnel: w461 -> [w487]
        tunnel: w453 -> [w489] mode=indexing
        shift-right: [w490] -> _
        shift-left: _ -> [w491]
        n162 = call "Cell color by inspection (2D).vi"("에러 입력(에러 없음)"=w491, "테이블 입력"=w489, "Spec"=w487) -> ("에러 출력"=w490:errorcluster, "Data(str)"=w488:string[][])  [unwired: 6 in, 1 out]
      }
      n163 = Index Array(array=w476) -> (element #1=w475:string[][], element #2=w474:string[][])  [unwired: 6 in]
      n164 = Transpose 2D Array(2D array=w450) -> (transposed array=w468:string[][])
      n165 = Insert Into Array(array=w468, index (col)=0 ("비활성화된 인덱스 (열)"), new element=w451) -> (w466:string[][])  [unwired: 1 in]
      n166 = Index Array(array=w460) -> (element #1=w459:string[][], element #2=w456:string[][])  [unwired: 6 in]
      n167 = call "Variables Data IO.vi"("Write blank data ?(F)"=w447, "Select"=Cmd_Var_Data_IO."Result2", "error in"=w478, "Data In"=w474, "Func_ext"=w477) -> ("error out"=w464:errorcluster, "Func_ext Out"=w465:string)  [unwired: 4 in, 1 out]
      n168 = call "Variables Data IO.vi"("Select"=Cmd_Var_Data_IO."Result_Temp", "error in"=w464, "Data In"=w466, "Func_ext"=w465) -> ("error out"=w462:errorcluster, "Func_ext Out"=w463:string)  [unwired: 5 in, 1 out]
      n169 = call "Variables Data IO.vi"("Write blank data ?(F)"=w447, "Select"=Cmd_Var_Data_IO."Result3", "error in"=w462, "Data In"=w473, "Func_ext"=w463) -> ("error out"=w449:errorcluster, "Func_ext Out"=w457:string)  [unwired: 4 in, 1 out]
      n170 = call "Variables Data IO.vi"("Write blank data ?(F)"=w447, "Select"=Cmd_Var_Data_IO."Result_ADJ2", "error in"=w449, "Data In"=w456, "Func_ext"=w457) -> ("error out"=w448:errorcluster)  [unwired: 4 in, 2 out]
    }
    frame "Length_13" {
      w554 = TRUE ("Write blank data ?(T)")
      # "INS_1=MEAS, EX_1=MEAS2, EX_2=MEAS3"
      n171 = Index Array(array=w560) -> (element=w537:refnum<vi>)  [unwired: 1 in]
      n172 = Index Array(array=w551) -> (element #1=w550:refnum<vi>, element #2=w546:refnum<vi>)  [unwired: 2 in]
      n173 = Unbundle By Name(w552) -> ("숫자형 3"=w532:dbl)
      n174 = property class="Tbl (엄격한)"(reference=w550) -> ("Value"=w547:string[][])  [unwired: 1 in, 2 out]
      n175 = property class="Tbl (엄격한)"(reference=w546) -> ("Value"=w545:string[][])  [unwired: 1 in, 2 out]
      n176 = Array Subset(array=w544, index (col)=0 ("인덱스"), length (col)=2 ("길이")) -> (w535:string[][])  [unwired: 2 in]
      n177 = call "Variables Data IO.vi"("Write blank data ?(F)"=w554, "Select"=Cmd_Var_Data_IO."Result2", "error in"=w559, "Data In"=w547, "Func_ext"=w557) -> ("error out"=w556:errorcluster, "Func_ext Out"=w555:string)  [unwired: 4 in, 1 out]
      n178 = call "Variables Data IO.vi"("Write blank data ?(F)"=w554, "Select"=Cmd_Var_Data_IO."Result3", "error in"=w556, "Data In"=w545, "Func_ext"=w555) -> ("error out"=w538:errorcluster)  [unwired: 4 in, 2 out]
      n179 = property class="Tbl (엄격한)"(reference=w537, error in=w538) -> (reference out=w542:refnum<vi>, error out=w541:errorcluster, "DisabledEnum"=w543:T4, "Value"=w534:string[][])
      n180 = Fract/Exp String To Number(string=w535) -> (number=w540:dbl[][])  [unwired: 3 in, 1 out]
      n181 = Fract/Exp String To Number(string=w534) -> (number=w539:dbl[][])  [unwired: 3 in, 1 out]
      n182 = Subtract(x=w540, y=w532) -> (x-y=w533:dbl[][])
      n183 = case shown="\"Enabled\"" w543 {
        tunnel: [w566 w574] -> w536
        tunnel: w539 -> [w565 _]
        tunnel: w533 -> [w564 _]
        tunnel: w541 -> [w563 w574]
        tunnel: w542 -> [w562 _]
        tunnel: w534 -> [w561 _]
        frame "Enabled" {
          n184 = for {
            tunnel: w564 -> [w568] mode=indexing
            tunnel: w565 -> [w569] mode=indexing
            tunnel: w562 -> [w570]
            tunnel: w561 -> [w571] mode=indexing
            shift-right: [w572] -> w566
            shift-left: w563 -> [w573]
            i -> [w567]
            n185 = call "Cell color by inspection (1D).vi"("행번호"=w567, "Spec"=w568, "Data (DBL)"=w569, "에러 입력"=w573, "테이블 입력"=w570, "Data (str)"=w571) -> ("에러 출력"=w572:errorcluster)  [unwired: 5 in]
          }
        }
        frame Default {
        }
      }
    }
    frame "Length_14" {
      n186 = Array Subset(array=w581, index (col)=0 ("인덱스"), length (col)=2 ("길이")) -> (w575:string[][])  [unwired: 2 in]
      n187 = for {
        tunnel: w580 -> [w595] mode=indexing
        tunnel: w575 -> [w585]
        tunnel: [w593] -> w578 mode=concatenating
        shift-right: [w594] -> w579
        shift-left: w584 -> [w599]
        tunnel: w577 -> [w592] mode=indexing
        tunnel: [w587] -> w576 mode=indexing
        n188 = property class="Tbl (엄격한)"(reference=w592) -> ("Value"=w591:string[][])  [unwired: 1 in, 2 out]
        n189 = property class="Tbl (엄격한)"(reference=w595, error in=w599) -> (reference out=w598:refnum<vi>, error out=w597:errorcluster, "Value"=w593:string[][])
        n190 = Index Array(array=w591, index (col)=5 ("비활성화된 인덱스 (열)")) -> (element=w589:string[])  [unwired: 1 in]
        n191 = Fract/Exp String To Number(string=w585) -> (number=w588:dbl[][])  [unwired: 3 in, 1 out]
        n192 = Fract/Exp String To Number(string=w593) -> (number=w596:dbl[][])  [unwired: 3 in, 1 out]
        n193 = Fract/Exp String To Number(string=w589) -> (number=w586:dbl[])  [unwired: 3 in, 1 out]
        n194 = for {
          tunnel: w588 -> [w603] mode=indexing
          tunnel: w596 -> [w605] mode=indexing
          tunnel: w598 -> [w606]
          tunnel: w593 -> [w607] mode=indexing
          shift-right: [w608] -> w594
          shift-left: w597 -> [w609]
          tunnel: w586 -> [w600] mode=indexing
          tunnel: [w601] -> w587 mode=indexing
          i -> [w604]
          n195 = Add(x=w603, y=w600) -> (x+y=w602:dbl[])
          n196 = call "Cell color by inspection (1D).vi"("행번호"=w604, "Spec"=w602, "Data (DBL)"=w605, "에러 입력"=w609, "테이블 입력"=w606, "Data (str)"=w607) -> ("에러 출력"=w608:errorcluster)  [unwired: 5 in]
          n197 = Build Array (concatenate)(w602, w600) -> (w601:dbl[])
        }
      }
    }
    frame "Length_15" {
      w611 = 0.0
      # "GH_zb"
      # "GH_za"
      # "FE_zb"
      # "FE_za"
      # "zb"
      # "za"
      n198 = Index Array(array=w648) -> (element=w645:refnum<vi>)  [unwired: 1 in]
      n199 = Unbundle By Name(w637) -> ("문자배열 2D"=w636:string[][])
      n200 = property class="Tbl (엄격한)"(reference=w645, error in=w641) -> (error out=w640:errorcluster, "Value"=w639:string[][])  [unwired: 1 out]
      n201 = Array Subset(array=w650, index (col)=0 ("인덱스"), length (col)=2 ("길이")) -> (w647:string[][])  [unwired: 2 in]
      n202 = Index Array(array=w649) -> (element #1=w646:refnum<vi>, element #2=w616:refnum<vi>)  [unwired: 2 in]
      n203 = call "Variables Data IO.vi"("Write blank data ?(F)"=TRUE ("Write blank data ?"), "Select"=Cmd_Var_Data_IO."Result2", "error in"=w640, "Data In"=w639, "Func_ext"=w638) -> ("error out"=w642:errorcluster)  [unwired: 4 in, 2 out]
      n204 = Fract/Exp String To Number(string=w647) -> (number=w617:dbl[][])  [unwired: 3 in, 1 out]
      n205 = property class="Tbl (엄격한)"(reference=w646, error in=w642) -> (error out=w632:errorcluster, "Value"=w610:string[][])  [unwired: 1 out]
      n206 = Fract/Exp String To Number(string=w636) -> (number=w635:dbl[][])  [unwired: 3 in, 1 out]
      n207 = Index Array(array=w635, index (col) #1=5 ("비활성화된 인덱스 (열)"), index (col) #2=4 ("비활성화된 인덱스 (열)")) -> (element #1=w627:dbl[], element #2=w631:dbl[])  [unwired: 2 in]
      n208 = Transpose 2D Array(2D array=w610) -> (transposed array=w615:string[][])
      n209 = Fract/Exp String To Number(string=w615) -> (number=w621:dbl[][])  [unwired: 3 in, 1 out]
      n210 = Index Array(array=w627) -> (element #1=w625:dbl, element #2=w626:dbl, element #3=w629:dbl)  [unwired: 3 in]
      n211 = Index Array(array=w631) -> (element #1=w623:dbl, element #2=w624:dbl, element #3=w630:dbl)  [unwired: 3 in]
      n212 = for {
        tunnel: w621 -> [w684] mode=indexing
        tunnel: 4.85e-06 ("C") -> [w685]
        tunnel: w629 -> [w683]
        shift-right: [w675] -> w620
        shift-left: w632 -> [w682]
        tunnel: w630 -> [w678]
        tunnel: w626 -> [w680]
        tunnel: w625 -> [w679]
        tunnel: w624 -> [w677]
        tunnel: w623 -> [w676]
        tunnel: [w672] -> w618 mode=indexing
        tunnel: w615 -> [w674] mode=indexing
        tunnel: [w673] -> w614 mode=indexing
        shift-right: [w671] -> _
        shift-left: w611 -> [w670]
        shift-right: [w669] -> _
        shift-left: w611 -> [w668]
        shift-right: [w665] -> _
        shift-left: w611 -> [w667]
        shift-right: [w663] -> _
        shift-left: w611 -> [w666]
        shift-right: [w664] -> _
        shift-left: w611 -> [w662]
        shift-right: [w660] -> _
        shift-left: w611 -> [w661]
        i -> [w681]
        n213 = case shown="4" w681 {
          tunnel: w685 -> [w708 w772 w835 w904 w973 w1041 w1107 w1171]
          tunnel: w684 -> [w706 w770 w833 w902 w971 w1039 w1105 w1169]
          tunnel: w683 -> [w704 w768 _ _ _ _ _ _]
          tunnel: [w698 w762 w830 w899 w968 w1036 w1102 w1166] -> w672
          tunnel: [w697 w761 w829 w898 w967 w1035 w1101 w1165] -> w675
          tunnel: w682 -> [w696 w760 w828 w897 w966 w1034 w1100 w1164]
          tunnel: w680 -> [_ _ _ _ w953 w1020 _ w1154]
          tunnel: w679 -> [_ _ w821 w892 _ _ w1095 _]
          tunnel: w678 -> [w694 w758 _ _ _ _ _ _]
          tunnel: w677 -> [_ _ _ _ w954 w1021 _ w1153]
          tunnel: w676 -> [_ _ w824 w893 _ _ w1096 _]
          tunnel: w674 -> [w693 w757 w826 w895 w965 w1032 w1098 w1162]
          tunnel: [w692 w756 w825 w894 w964 w1031 w1097 w1161] -> w673
          tunnel: [w691 w754 w823 w884 w963 w1030 w1092 w1160] -> w671
          tunnel: w670 -> [_ w754 w822 w884 w962 w1029 w1092 w1160]
          tunnel: [w690 w755 w822 w883 w962 w1029 w1091 w1159] -> w669
          tunnel: w668 -> [w690 _ w823 w883 w963 w1030 w1091 w1159]
          tunnel: w667 -> [w689 w753 w815 w887 _ w1025 w1089 w1157]
          tunnel: w666 -> [w688 w752 w816 w888 w955 _ w1090 w1158]
          tunnel: [w689 w753 w815 w887 w956 w1025 w1089 w1157] -> w665
          tunnel: [w686 w750 w817 w885 w958 w1024 w1094 w1156] -> w664
          tunnel: [w688 w752 w816 w888 w955 w1022 w1090 w1158] -> w663
          tunnel: w662 -> [w686 w750 _ w885 w958 w1024 w1094 w1156]
          tunnel: [w687 w751 w814 w886 w957 w1023 w1093 w1155] -> w660
          tunnel: w661 -> [w687 w751 w814 _ w957 w1023 w1093 w1155]
          frame 0, Default {
            # "대각선방향 (AC)"
            n214 = for {
              tunnel: w706 -> [w710] mode=indexing
              shift-right: [w709] -> _
              shift-left: 0.0 -> [w711]
              tunnel: [w709] -> w705 mode=indexing
              n215 = Add(x=w711, y=w710) -> (x+y=w709:dbl)
            }
            n216 = Divide(x=w704, y=2.0) -> (x/y=w702:dbl)
            n217 = To Long Integer(number=w704) -> (32bit integer=w695:i32)
            n218 = To Long Integer(number=w702) -> (32bit integer=w701:i32)
            n219 = Index Array(array=w705, index #1=w695, index #2=w701) -> (element #1=w700:dbl, element #2=w699:dbl)
            n220 = for {
              tunnel: w708 -> [w729]
              tunnel: w695 -> [w728]
              tunnel: w705 -> [w726] mode=indexing
              tunnel: w700 -> [w725]
              tunnel: w699 -> [w724]
              tunnel: [w713] -> w698 mode=indexing
              shift-right: [w722] -> w697
              shift-left: w696 -> [w721]
              tunnel: w694 -> [w712]
              tunnel: w693 -> [w720] mode=indexing
              tunnel: [w714] -> w692 mode=indexing
              tunnel: [w713] -> w691
              i -> [w727]
              w718 = "ⅹ" ("y")
              n221 = xnode "수식"("에러 입력(에러 없음)"=w721, "ym"=w726, "m"=w727, "yN"=w725, "yN2"=w724, "N"=w728, "C"=w729, "F"=w712) -> ("결과"=w716:dbl, "에러 출력"=w722:errorcluster)
              n222 = Equal?(x=w718, y=w720) -> (x = y?=w719:bool)
              n223 = call "DBL Round.vi"("반올림자리수"=2, "DBL in"=w716) -> ("DBL out"=w713:dbl)  [unwired: 1 in]
              n224 = Number To Fractional String(number=w713, precision (6)=i16 1 ("정밀도(6)")) -> (F-format string=w715:string)  [unwired: 2 in]
              n225 = Select(t=w718, s=w719, f=w715) -> (s? t:f=w714:string)
            }
          }
          frame 1 {
            # "대각선방향 (BD)"
            n226 = for {
              tunnel: w770 -> [w774] mode=indexing
              shift-right: [w773] -> _
              shift-left: 0.0 -> [w775]
              tunnel: [w773] -> w769 mode=indexing
              n227 = Add(x=w775, y=w774) -> (x+y=w773:dbl)
            }
            n228 = Divide(x=w768, y=2.0) -> (x/y=w766:dbl)
            n229 = To Long Integer(number=w768) -> (32bit integer=w759:i32)
            n230 = To Long Integer(number=w766) -> (32bit integer=w765:i32)
            n231 = Index Array(array=w769, index #1=w759, index #2=w765) -> (element #1=w764:dbl, element #2=w763:dbl)
            n232 = for {
              tunnel: w772 -> [w793]
              tunnel: w759 -> [w792]
              tunnel: w769 -> [w790] mode=indexing
              tunnel: w764 -> [w789]
              tunnel: w763 -> [w788]
              tunnel: [w777] -> w762 mode=indexing
              shift-right: [w786] -> w761
              shift-left: w760 -> [w785]
              tunnel: w758 -> [w776]
              tunnel: w757 -> [w784] mode=indexing
              tunnel: [w778] -> w756 mode=indexing
              tunnel: [w777] -> w755
              i -> [w791]
              w782 = "ⅹ" ("y")
              n233 = xnode "수식"("에러 입력(에러 없음)"=w785, "ym"=w790, "m"=w791, "yN"=w789, "yN2"=w788, "N"=w792, "C"=w793, "F"=w776) -> ("결과"=w780:dbl, "에러 출력"=w786:errorcluster)
              n234 = Equal?(x=w782, y=w784) -> (x = y?=w783:bool)
              n235 = call "DBL Round.vi"("반올림자리수"=2, "DBL in"=w780) -> ("DBL out"=w777:dbl)  [unwired: 1 in]
              n236 = Number To Fractional String(number=w777, precision (6)=i16 1 ("정밀도(6)")) -> (F-format string=w779:string)  [unwired: 2 in]
              n237 = Select(t=w782, s=w783, f=w779) -> (s? t:f=w778:string)
            }
          }
          frame 2 {
            # "가로 (AB)"
            n238 = for {
              tunnel: w833 -> [w838] mode=indexing
              shift-right: [w837] -> _
              shift-left: 0.0 -> [w839]
              tunnel: [w837] -> w832 mode=indexing
              tunnel: [w836] -> _
              i -> [w836]
              n239 = Add(x=w839, y=w838) -> (x+y=w837:dbl)
            }
            n240 = Divide(x=w821, y=2.0) -> (x/y=w819:dbl)
            n241 = To Long Integer(number=w819) -> (32bit integer=w818:i32)
            n242 = To Long Integer(number=w821) -> (32bit integer=w827:i32)
            n243 = Index Array(array=w832, index=w827) -> (element=w831:dbl)
            n244 = for {
              tunnel: w835 -> [w860]
              tunnel: w827 -> [w859]
              tunnel: w832 -> [w858] mode=indexing
              tunnel: w831 -> [w857]
              tunnel: w822 -> [w856]
              tunnel: [w842] -> w830 mode=indexing
              shift-right: [w854] -> w829
              shift-left: w828 -> [w853]
              tunnel: w824 -> [w840]
              tunnel: w826 -> [w852] mode=indexing
              tunnel: [w848] -> w825 mode=indexing
              tunnel: w823 -> [w847]
              tunnel: w818 -> [w843]
              tunnel: [w842] -> w817 if=w841
              i -> [w844]
              w850 = "ⅹ" ("y")
              n245 = xnode "수식"("에러 입력(에러 없음)"=w853, "ym"=w858, "yN'"=w857, "N'"=w859, "C"=w860, "F"=w840, "za"=w856, "zb"=w847, "m"=w844) -> ("결과"=w849:dbl, "에러 출력"=w854:errorcluster)
              n246 = Equal?(x=w844, y=w843) -> (x = y?=w841:bool)
              n247 = Equal?(x=w850, y=w852) -> (x = y?=w851:bool)
              n248 = call "DBL Round.vi"("반올림자리수"=2, "DBL in"=w849) -> ("DBL out"=w842:dbl)  [unwired: 1 in]
              n249 = Number To Fractional String(number=w842, precision (6)=i16 1 ("정밀도(6)")) -> (F-format string=w846:string)  [unwired: 2 in]
              n250 = Select(t=w850, s=w851, f=w846) -> (s? t:f=w848:string)
            }
          }
          frame 3 {
            # "가로 (DC)"
            n251 = for {
              tunnel: w902 -> [w907] mode=indexing
              shift-right: [w906] -> _
              shift-left: 0.0 -> [w908]
              tunnel: [w906] -> w901 mode=indexing
              tunnel: [w905] -> _
              i -> [w905]
              n252 = Add(x=w908, y=w907) -> (x+y=w906:dbl)
            }
            n253 = Divide(x=w892, y=2.0) -> (x/y=w890:dbl)
            n254 = To Long Integer(number=w890) -> (32bit integer=w889:i32)
            n255 = To Long Integer(number=w892) -> (32bit integer=w896:i32)
            n256 = Index Array(array=w901, index=w896) -> (element=w900:dbl)
            n257 = for {
              tunnel: w904 -> [w929]
              tunnel: w896 -> [w928]
              tunnel: w901 -> [w927] mode=indexing
              tunnel: w900 -> [w926]
              tunnel: w884 -> [w925]
              tunnel: [w911] -> w899 mode=indexing
              shift-right: [w923] -> w898
              shift-left: w897 -> [w922]
              tunnel: w893 -> [w909]
              tunnel: w895 -> [w921] mode=indexing
              tunnel: [w917] -> w894 mode=indexing
              tunnel: w883 -> [w916]
              tunnel: w889 -> [w912]
              tunnel: [w911] -> w886 if=w910
              i -> [w913]
              w919 = "ⅹ" ("y")
              n258 = xnode "수식"("에러 입력(에러 없음)"=w922, "ym"=w927, "yN'"=w926, "N'"=w928, "C"=w929, "F"=w909, "za"=w925, "zb"=w916, "m"=w913) -> ("결과"=w918:dbl, "에러 출력"=w923:errorcluster)
              n259 = Equal?(x=w913, y=w912) -> (x = y?=w910:bool)
              n260 = Equal?(x=w919, y=w921) -> (x = y?=w920:bool)
              n261 = call "DBL Round.vi"("반올림자리수"=2, "DBL in"=w918) -> ("DBL out"=w911:dbl)  [unwired: 1 in]
              n262 = Number To Fractional String(number=w911, precision (6)=i16 1 ("정밀도(6)")) -> (F-format string=w915:string)  [unwired: 2 in]
              n263 = Select(t=w919, s=w920, f=w915) -> (s? t:f=w917:string)
            }
          }
          frame 4 {
            # "세로 (AD)"
            n264 = Divide(x=w953, y=2.0) -> (x/y=w960:dbl)
            n265 = for {
              tunnel: w971 -> [w975] mode=indexing
              shift-right: [w974] -> _
              shift-left: 0.0 -> [w976]
              tunnel: [w974] -> w970 mode=indexing
              n266 = Add(x=w976, y=w975) -> (x+y=w974:dbl)
            }
            n267 = To Long Integer(number=w960) -> (32bit integer=w959:i32)
            n268 = To Long Integer(number=w953) -> (32bit integer=w952:i32)
            n269 = Index Array(array=w970, index=w952) -> (element=w969:dbl)
            n270 = for {
              tunnel: w973 -> [w997]
              tunnel: w952 -> [w996]
              tunnel: w970 -> [w995] mode=indexing
              tunnel: w969 -> [w994]
              tunnel: w962 -> [w979]
              tunnel: [w981] -> w968 mode=indexing
              shift-right: [w992] -> w967
              shift-left: w966 -> [w991]
              tunnel: w954 -> [w977]
              tunnel: w965 -> [w990] mode=indexing
              tunnel: [w986] -> w964 mode=indexing
              tunnel: w963 -> [w978]
              tunnel: w959 -> [w982]
              tunnel: [w981] -> w956 if=w980
              i -> [w983]
              w988 = "ⅹ" ("y")
              n271 = xnode "수식"("에러 입력(에러 없음)"=w991, "ym"=w995, "yN'"=w994, "N'"=w996, "C"=w997, "F"=w977, "za"=w978, "zb"=w979, "m"=w983) -> ("결과"=w987:dbl, "에러 출력"=w992:errorcluster)
              n272 = Equal?(x=w983, y=w982) -> (x = y?=w980:bool)
              n273 = Equal?(x=w988, y=w990) -> (x = y?=w989:bool)
              n274 = call "DBL Round.vi"("반올림자리수"=2, "DBL in"=w987) -> ("DBL out"=w981:dbl)  [unwired: 1 in]
              n275 = Number To Fractional String(number=w981, precision (6)=i16 1 ("정밀도(6)")) -> (F-format string=w985:string)  [unwired: 2 in]
              n276 = Select(t=w988, s=w989, f=w985) -> (s? t:f=w986:string)
            }
          }
          frame 5 {
            # "세로 (BC)"
            n277 = for {
              tunnel: w1039 -> [w1044] mode=indexing
              shift-right: [w1043] -> _
              shift-left: 0.0 -> [w1045]
              tunnel: [w1043] -> w1038 mode=indexing
              tunnel: [w1042] -> _
              i -> [w1042]
              n278 = Add(x=w1045, y=w1044) -> (x+y=w1043:dbl)
            }
            n279 = Divide(x=w1020, y=2.0) -> (x/y=w1027:dbl)
            n280 = To Long Integer(number=w1027) -> (32bit integer=w1026:i32)
            n281 = To Long Integer(number=w1020) -> (32bit integer=w1033:i32)
            n282 = Index Array(array=w1038, index=w1033) -> (element=w1037:dbl)
            n283 = for {
              tunnel: w1041 -> [w1066]
              tunnel: w1033 -> [w1065]
              tunnel: w1038 -> [w1064] mode=indexing
              tunnel: w1037 -> [w1063]
              tunnel: w1029 -> [w1046]
              tunnel: [w1050] -> w1036 mode=indexing
              shift-right: [w1061] -> w1035
              shift-left: w1034 -> [w1060]
              tunnel: w1021 -> [w1048]
              tunnel: w1032 -> [w1059] mode=indexing
              tunnel: [w1055] -> w1031 mode=indexing
              tunnel: w1030 -> [w1047]
              tunnel: w1026 -> [w1051]
              tunnel: [w1050] -> w1022 if=w1049
              i -> [w1052]
              w1057 = "ⅹ" ("y")
              n284 = xnode "수식"("에러 입력(에러 없음)"=w1060, "ym"=w1064, "yN'"=w1063, "N'"=w1065, "C"=w1066, "F"=w1048, "za"=w1047, "zb"=w1046, "m"=w1052) -> ("결과"=w1056:dbl, "에러 출력"=w1061:errorcluster)
              n285 = Equal?(x=w1052, y=w1051) -> (x = y?=w1049:bool)
              n286 = Equal?(x=w1057, y=w1059) -> (x = y?=w1058:bool)
              n287 = call "DBL Round.vi"("반올림자리수"=2, "DBL in"=w1056) -> ("DBL out"=w1050:dbl)  [unwired: 1 in]
              n288 = Number To Fractional String(number=w1050, precision (6)=i16 1 ("정밀도(6)")) -> (F-format string=w1054:string)  [unwired: 2 in]
              n289 = Select(t=w1057, s=w1058, f=w1054) -> (s? t:f=w1055:string)
            }
          }
          frame 6 {
            # "중앙 (FE)"
            n290 = for {
              tunnel: w1105 -> [w1110] mode=indexing
              shift-right: [w1109] -> _
              shift-left: 0.0 -> [w1111]
              tunnel: [w1109] -> w1104 mode=indexing
              tunnel: [w1108] -> _
              i -> [w1108]
              n291 = Add(x=w1111, y=w1110) -> (x+y=w1109:dbl)
            }
            n292 = To Long Integer(number=w1095) -> (32bit integer=w1099:i32)
            n293 = Index Array(array=w1104, index=w1099) -> (element=w1103:dbl)
            n294 = for {
              tunnel: w1107 -> [w1130]
              tunnel: w1099 -> [w1129]
              tunnel: w1104 -> [w1128] mode=indexing
              tunnel: w1103 -> [w1127]
              tunnel: w1089 -> [w1126]
              tunnel: [w1113] -> w1102 mode=indexing
              shift-right: [w1124] -> w1101
              shift-left: w1100 -> [w1123]
              tunnel: w1096 -> [w1112]
              tunnel: w1098 -> [w1122] mode=indexing
              tunnel: [w1118] -> w1097 mode=indexing
              tunnel: w1090 -> [w1117]
              i -> [w1114]
              w1120 = "ⅹ" ("y")
              n295 = xnode "수식"("에러 입력(에러 없음)"=w1123, "ym"=w1128, "yN'"=w1127, "N'"=w1129, "C"=w1130, "F"=w1112, "za"=w1126, "zb"=w1117, "m"=w1114) -> ("결과"=w1119:dbl, "에러 출력"=w1124:errorcluster)
              n296 = Equal?(x=w1120, y=w1122) -> (x = y?=w1121:bool)
              n297 = call "DBL Round.vi"("반올림자리수"=2, "DBL in"=w1119) -> ("DBL out"=w1113:dbl)  [unwired: 1 in]
              n298 = Number To Fractional String(number=w1113, precision (6)=i16 1 ("정밀도(6)")) -> (F-format string=w1116:string)  [unwired: 2 in]
              n299 = Select(t=w1120, s=w1121, f=w1116) -> (s? t:f=w1118:string)
            }
          }
          frame 7 {
            # "중앙 (GH)"
            n300 = for {
              tunnel: w1169 -> [w1174] mode=indexing
              shift-right: [w1173] -> _
              shift-left: 0.0 -> [w1175]
              tunnel: [w1173] -> w1168 mode=indexing
              tunnel: [w1172] -> _
              i -> [w1172]
              n301 = Add(x=w1175, y=w1174) -> (x+y=w1173:dbl)
            }
            n302 = To Long Integer(number=w1154) -> (32bit integer=w1163:i32)
            n303 = Index Array(array=w1168, index=w1163) -> (element=w1167:dbl)
            n304 = for {
              tunnel: w1171 -> [w1194]
              tunnel: w1163 -> [w1193]
              tunnel: w1168 -> [w1192] mode=indexing
              tunnel: w1167 -> [w1191]
              tunnel: w1156 -> [w1190]
              tunnel: [w1177] -> w1166 mode=indexing
              shift-right: [w1188] -> w1165
              shift-left: w1164 -> [w1187]
              tunnel: w1153 -> [w1176]
              tunnel: w1162 -> [w1186] mode=indexing
              tunnel: [w1182] -> w1161 mode=indexing
              tunnel: w1155 -> [w1181]
              i -> [w1178]
              w1184 = "ⅹ" ("y")
              n305 = xnode "수식"("에러 입력(에러 없음)"=w1187, "ym"=w1192, "yN'"=w1191, "N'"=w1193, "C"=w1194, "F"=w1176, "za"=w1190, "zb"=w1181, "m"=w1178) -> ("결과"=w1183:dbl, "에러 출력"=w1188:errorcluster)
              n306 = Equal?(x=w1184, y=w1186) -> (x = y?=w1185:bool)
              n307 = call "DBL Round.vi"("반올림자리수"=2, "DBL in"=w1183) -> ("DBL out"=w1177:dbl)  [unwired: 1 in]
              n308 = Number To Fractional String(number=w1177, precision (6)=i16 1 ("정밀도(6)")) -> (F-format string=w1180:string)  [unwired: 2 in]
              n309 = Select(t=w1184, s=w1185, f=w1180) -> (s? t:f=w1182:string)
            }
          }
        }
      }
      n310 = Transpose 2D Array(2D array=w614) -> (transposed array=w612:string[][])
      n311 = Transpose 2D Array(2D array=w618) -> (transposed array=w613:dbl[][])
      n312 = for {
        tunnel: w617 -> [w656] mode=indexing
        tunnel: w613 -> [w657] mode=indexing
        shift-right: [w658] -> w619
        shift-left: w620 -> [w659]
        tunnel: w616 -> [w654]
        tunnel: w612 -> [w653] mode=indexing
        i -> [w655]
        n313 = call "Cell color by inspection (1D).vi"("행번호"=w655, "Spec"=w656, "Data (DBL)"=w657, "에러 입력"=w659, "테이블 입력"=w654, "Data (str)"=w653) -> ("에러 출력"=w658:errorcluster)  [unwired: 5 in]
      }
      n314 = property class="Tbl (엄격한)"(reference=w616, error in=w619, "Value"=w612) -> (error out=w622:errorcluster)  [unwired: 1 out]
    }
    frame "Length_2" {
      w1236 = TRUE ("Write blank data ?(T)")
      # "INS_1=MEAS, EX_1=MEAS2, EX_2=MEAS3"
      n315 = Index Array(array=w1243) -> (element=w1224:refnum<vi>)  [unwired: 1 in]
      n316 = Unbundle By Name(w1233) -> ("불리언 1D"=w1232:bool[])
      n317 = Array Subset(array=w1240, index (col)=0 ("인덱스"), length (col)=2 ("길이")) -> (w1225:string[][])  [unwired: 2 in]
      n318 = for {
        tunnel: w1232 -> [w1247] mode=indexing
        tunnel: [w1249] -> w1231 mode=indexing
        tunnel: w1229 -> [w1248] mode=indexing
        tunnel: [w1245] -> w1228 mode=indexing
        n319 = property class="Tbl (엄격한)"(reference=w1248) -> ("Value"=w1246:string[][])  [unwired: 1 in, 2 out]
        n320 = Format Into String(w1247) -> (resulting string=w1249:string)  [unwired: 3 in, 1 out]
        n321 = Select(t=w1246, s=w1247, f=string[][] []) -> (s? t:f=w1245:string[][])
      }
      n322 = Build Array(w1231) -> (w1230:string[][])
      n323 = Index Array(array=w1228) -> (element #1=w1227:string[][], element #2=w1226:string[][])  [unwired: 6 in]
      n324 = call "Variables Data IO.vi"("Select"=Cmd_Var_Data_IO."Result_Temp", "error in"=w1221, "Data In"=w1230, "Func_ext"=w1220) -> ("error out"=w1218:errorcluster, "Func_ext Out"=w1219:string)  [unwired: 5 in, 1 out]
      n325 = call "Variables Data IO.vi"("Write blank data ?(F)"=w1236, "Select"=Cmd_Var_Data_IO."Result2", "error in"=w1218, "Data In"=w1227, "Func_ext"=w1219) -> ("error out"=w1238:errorcluster, "Func_ext Out"=w1237:string)  [unwired: 4 in, 1 out]
      n326 = call "Variables Data IO.vi"("Write blank data ?(F)"=w1236, "Select"=Cmd_Var_Data_IO."Result3", "error in"=w1238, "Data In"=w1226, "Func_ext"=w1237) -> ("error out"=w1217:errorcluster)  [unwired: 4 in, 2 out]
      n327 = call "Cell color by inspection (2D).vi"("에러 입력(에러 없음)"=w1217, "테이블 입력"=w1224, "Spec"=w1225) -> ("에러 출력"=w1222:errorcluster, "Data(str)"=w1223:string[][])  [unwired: 6 in, 1 out]
    }
    frame "Length_3" {
      w1274 = TRUE ("Write blank data ?(T)")
      # "INS_1=MEAS, INS_2=ADJ, EX_1=MEAS2"
      n328 = Index Array(array=w1270) -> (element=w1269:refnum<vi>)  [unwired: 1 in]
      n329 = Array Subset(array=w1265, index (col)=0 ("인덱스"), length (col)=2 ("길이")) -> (w1259:string[][])  [unwired: 2 in]
      n330 = property class="Tbl (엄격한)"(reference=w1269) -> ("DisabledEnum"=w1252:T4, "Visible"=w1251:bool, "Value"=w1268:string[][])  [unwired: 1 in, 2 out]
      n331 = Unbundle By Name(w1272) -> ("문자열 1"=w1271:string)
      n332 = Equal?(x=T4."Enabled" ("비활성화"), y=w1252) -> (x = y?=w1254:bool)
      n333 = And(x=w1254, y=w1251) -> (x .and. y?=w1250:bool)
      n334 = Build Array(w1271) -> (w1264:string[])
      n335 = case shown="거짓" w1250 {
        tunnel: w1276 -> [w1278 w1285]
        tunnel: [w1278 w1284] -> w1275
        tunnel: w1274 -> [_ w1283]
        tunnel: w1268 -> [_ w1282]
        tunnel: w1258 -> [w1279 w1281]
        tunnel: [w1279 w1280] -> w1255
        frame False {
        }
        frame True {
          n336 = call "Variables Data IO.vi"("Write blank data ?(F)"=w1283, "Select"=Cmd_Var_Data_IO."Result2", "error in"=w1281, "Data In"=w1282, "Func_ext"=w1285) -> ("error out"=w1280:errorcluster, "Func_ext Out"=w1284:string)  [unwired: 4 in, 1 out]
        }
      }
      n337 = Build Array(w1264) -> (w1263:string[][])
      n338 = call "Variables Data IO.vi"("Write blank data ?(F)"=w1274, "Select"=Cmd_Var_Data_IO."Result3", "error in"=w1255, "Data In"=w1263, "Func_ext"=w1275) -> ("error out"=w1257:errorcluster)  [unwired: 4 in, 2 out]
      n339 = for {
        tunnel: w1260 -> [w1291] mode=indexing
        tunnel: [w1287] -> w1277 mode=indexing
        tunnel: w1259 -> [w1288]
        shift-right: [w1289] -> w1256
        shift-left: w1257 -> [w1290]
        n340 = call "Cell color by inspection (2D).vi"("에러 입력(에러 없음)"=w1290, "테이블 입력"=w1291, "Spec"=w1288) -> ("에러 출력"=w1289:errorcluster, "Data(str)"=w1287:string[][])  [unwired: 6 in, 1 out]
      }
      n341 = Index Array(array=w1277) -> (element #1=w1262:string[][], element #2=w1261:string[][])  [unwired: 6 in]
    }
    frame "Length_4" {
      n342 = Index Array(array=w1313) -> (element=w1312:refnum<vi>)  [unwired: 1 in]
      n343 = Unbundle By Name(w1302) -> ("문자배열 2D"=w1299:string[][])
      n344 = Array Subset(array=w1306, index (col)=0 ("인덱스"), length (col)=2 ("길이")) -> (w1293:string[][])  [unwired: 2 in]
      n345 = call "Variables Data IO.vi"("Write blank data ?(F)"=TRUE ("Write blank data ?"), "Select"=Cmd_Var_Data_IO."Result2", "error in"=w1298, "Data In"=w1299, "Func_ext"=w1297) -> ("error out"=w1295:errorcluster, "Func_ext Out"=w1296:string)  [unwired: 4 in, 1 out]
      n346 = call "Variables Data IO.vi"("Select"=Cmd_Var_Data_IO."Condition", "error in"=w1295, "Func_ext"=w1296) -> ("error out"=w1305:errorcluster, "Data Out"=w1303:string[][])  [unwired: 6 in, 1 out]
      n347 = property class="Tbl (엄격한)"(reference=w1312, error in=w1305) -> (reference out=w1311:refnum<vi>, error out=w1309:errorcluster, "Value"=w1310:string[][], "DisabledEnum"=w1292:T4)
      n348 = case shown="\"Enabled\"" w1292 {
        tunnel: w1311 -> [w1325 _]
        tunnel: w1310 -> [w1324 _]
        tunnel: w1309 -> [w1323 w1336]
        tunnel: w1303 -> [w1322 _]
        tunnel: [w1315 w1336] -> w1294
        tunnel: w1293 -> [w1314 _]
        frame "Enabled" {
          n349 = Index Array(array=w1322, index (col)=0 ("비활성화된 인덱스 (열)")) -> (element=w1320:string[])  [unwired: 1 in]
          n350 = Fract/Exp String To Number(string=w1314) -> (number=w1326:dbl[][])  [unwired: 3 in, 1 out]
          n351 = Fract/Exp String To Number(string=w1320) -> (number=w1319:dbl[])  [unwired: 3 in, 1 out]
          n352 = Fract/Exp String To Number(string=w1324) -> (number=w1318:dbl[][])  [unwired: 3 in, 1 out]
          n353 = Divide(x=w1318, y=1000.0) -> (x/y=w1316:dbl[][])
          n354 = for {
            tunnel: w1326 -> [w1331] mode=indexing
            tunnel: w1316 -> [w1335] mode=indexing
            tunnel: w1325 -> [w1329]
            tunnel: w1324 -> [w1333] mode=indexing
            shift-right: [w1328] -> w1315
            shift-left: w1323 -> [w1330]
            tunnel: w1319 -> [w1334] mode=indexing
            i -> [w1327]
            n355 = Add(x=w1335, y=w1334) -> (x+y=w1332:dbl[])
            n356 = call "Cell color by inspection (1D).vi"("행번호"=w1327, "Spec"=w1331, "Data (DBL)"=w1332, "에러 입력"=w1330, "테이블 입력"=w1329, "Data (str)"=w1333) -> ("에러 출력"=w1328:errorcluster)  [unwired: 5 in]
          }
        }
        frame Default {
        }
      }
    }
    frame "Length_6_1" {
      n357 = Index Array(array=w1355) -> (element=w1344:refnum<vi>)  [unwired: 1 in]
      n358 = property class="Tbl (엄격한)"(reference=w1344, error in=w1353) -> (error out=w1341:errorcluster, "Value"=w1343:string[][])  [unwired: 1 out]
      n359 = Array Subset(array=w1358, index (col)=0 ("인덱스"), length (col)=2 ("길이")) -> (w1357:string[][])  [unwired: 2 in]
      n360 = Fract/Exp String To Number(string=w1357) -> (number=w1349:dbl[][])  [unwired: 3 in, 1 out]
      n361 = call "Variables Data IO.vi"("Write blank data ?(F)"=TRUE ("Write blank data ?(T)"), "Select"=Cmd_Var_Data_IO."Result3", "error in"=w1341, "Data In"=w1343, "Func_ext"=w1354) -> ("error out"=w1340:errorcluster, "Func_ext Out"=w1339:string)  [unwired: 4 in, 1 out]
      n362 = for {
        tunnel: [w1361] -> w1352 mode=indexing
        tunnel: w1349 -> [w1364]
        tunnel: w1356 -> [w1362] mode=indexing
        shift-right: [w1367] -> w1338
        shift-left: w1340 -> [w1363]
        n363 = property class="Tbl (엄격한)"(reference=w1362, error in=w1363) -> (reference out=w1366:refnum<vi>, error out=w1365:errorcluster, "Value"=w1361:string[][], "DisabledEnum"=w1360:T4)
        n364 = case shown="\"Enabled\"" w1360 {
          tunnel: [w1378 w1396] -> w1367
          tunnel: w1366 -> [w1377 _]
          tunnel: w1365 -> [w1376 w1396]
          tunnel: w1364 -> [w1375 _]
          tunnel: w1361 -> [w1373 _]
          frame "Enabled" {
            n365 = for {
              tunnel: w1373 -> [w1385] mode=indexing
              shift-right: [w1383] -> _
              shift-left: dbl[] [] -> [w1384]
              tunnel: [w1382] -> w1372 mode=indexing
              i -> [w1381]
              n366 = Fract/Exp String To Number(string=w1385) -> (number=w1383:dbl[])  [unwired: 3 in, 1 out]
              n367 = Quotient & Remainder(x=w1381, y=2) -> (x-y*floor(x/y)=w1379:i32)  [unwired: 1 out]
              n368 = case shown="기본" w1379 {
                tunnel: w1384 -> [_ w1388]
                tunnel: w1383 -> [_ w1387]
                tunnel: [_ w1386] -> w1382
                frame 0 {
                }
                frame Default {
                  n369 = Divide(x=w1387, y=w1388) -> (x/y=w1386:dbl[])
                }
              }
            }
            n370 = Delete From Array(array=w1372, index (row)=0 ("인덱스 (행)")) -> (deleted portion=w1369:dbl[], array with subset deleted=w1370:dbl[][])  [unwired: 2 in]
            n371 = Insert Into Array(array=w1370, new element=w1369) -> (w1368:dbl[][])  [unwired: 2 in]
            n372 = for {
              tunnel: w1375 -> [w1391] mode=indexing
              tunnel: w1368 -> [w1392] mode=indexing
              tunnel: w1377 -> [w1394]
              tunnel: w1373 -> [w1393] mode=indexing
              shift-right: [w1390] -> w1378
              shift-left: w1376 -> [w1395]
              i -> [w1389]
              n373 = call "Cell color by inspection (1D).vi"("행번호"=w1389, "Spec"=w1391, "Data (DBL)"=w1392, "에러 입력"=w1395, "테이블 입력"=w1394, "Data (str)"=w1393) -> ("에러 출력"=w1390:errorcluster)  [unwired: 5 in]
            }
          }
          frame Default {
          }
        }
      }
      n374 = Index Array(array=w1352) -> (element #1=w1359:string[][], element #2=w1342:string[][])  [unwired: 6 in]
      n375 = call "Variables Data IO.vi"("Write blank data ?(F)"=TRUE ("Write blank data ?(T)"), "Select"=Cmd_Var_Data_IO."Result2", "error in"=w1338, "Data In"=w1342, "Func_ext"=w1339) -> ("error out"=w1337:errorcluster)  [unwired: 4 in, 2 out]
    }
    frame "Length_7" {
      w1398 = TRUE ("Write blank data ?(T)")
      # "TBL_1_Check, TBL_n_na"
      n376 = Array Subset(array=w1413, index (col)=0 ("인덱스"), length (col)=2 ("길이")) -> (w1412:string[][])  [unwired: 2 in]
      n377 = case shown="\"10224-1\"" w1397 {
        tunnel: w1415 -> [w1426 w1430]
        tunnel: [w1417 w1428] -> w1414
        tunnel: w1412 -> [w1420 w1433]
        tunnel: w1411 -> [w1418 w1432]
        tunnel: w1410 -> [w1425 _]
        tunnel: [w1416 w1431] -> w1405
        tunnel: [w1423 w1427] -> w1403
        tunnel: [w1422 _] -> w1399
        frame Default {
          n378 = Index Array(array=w1426) -> (element #1=w1419:refnum<vi>, element #2=w1421:refnum<vi>)  [unwired: 2 in]
          n379 = Index Array(array=w1425) -> (element=w1424:refnum<vi>)  [unwired: 1 in]
          n380 = property class="Tbl (엄격한)"(reference=w1424) -> ("Value"=w1422:string[][])  [unwired: 1 in, 2 out]
          n381 = property class="Tbl (엄격한)"(reference=w1421) -> ("Value"=w1423:string[][])  [unwired: 1 in, 2 out]
          n382 = call "Cell color by inspection (2D).vi"("에러 입력(에러 없음)"=w1418, "테이블 입력"=w1419, "Spec"=w1420) -> ("에러 출력"=w1416:errorcluster, "Data(str)"=w1417:string[][])  [unwired: 6 in, 1 out]
        }
        frame "10224-1" {
          n383 = for {
            tunnel: [w1435] -> w1429 mode=indexing
            tunnel: w1433 -> [w1437]
            tunnel: w1430 -> [w1438] mode=indexing
            shift-right: [w1434] -> w1431
            shift-left: w1432 -> [w1436]
            n384 = call "Cell color by inspection (2D).vi"("에러 입력(에러 없음)"=w1436, "테이블 입력"=w1438, "Spec"=w1437) -> ("에러 출력"=w1434:errorcluster, "Data(str)"=w1435:string[][])  [unwired: 6 in, 1 out]
          }
          n385 = Index Array(array=w1429) -> (element #1=w1428:string[][], element #2=w1427:string[][])  [unwired: 6 in]
        }
      }
      n386 = call "Variables Data IO.vi"("Write blank data ?(F)"=w1398, "Select"=Cmd_Var_Data_IO."Result2", "error in"=w1405, "Data In"=w1403, "Func_ext"=w1409) -> ("error out"=w1400:errorcluster, "Func_ext Out"=w1401:string)  [unwired: 4 in, 1 out]
      n387 = call "Variables Data IO.vi"("Write blank data ?(F)"=w1398, "Select"=Cmd_Var_Data_IO."Result3", "error in"=w1400, "Data In"=w1399, "Func_ext"=w1401) -> ("error out"=w1408:errorcluster)  [unwired: 4 in, 2 out]
    }
    frame "Length_9" {
      # "TBL_1_Check"
      n388 = for {
        tunnel: w1444 -> [w1449] mode=indexing
        tunnel: w1442 -> [w1453] mode=indexing
        shift-right: [w1446] -> w1443
        shift-left: w1441 -> [w1452]
        tunnel: [w1447] -> w1440 mode=indexing
        n389 = property class="Tbl (엄격한)"(reference=w1453, error in=w1452) -> (error out=w1448:errorcluster, "Value"=w1451:string[][])  [unwired: 1 out]
        n390 = Delete From Array(array=w1451, index (col)=2 ("비활성화된 인덱스 (열)")) -> (array with subset deleted=w1445:string[][])  [unwired: 2 in, 1 out]
        n391 = call "Cell color by inspection (2D).vi"("에러 입력(에러 없음)"=w1448, "테이블 입력"=w1449, "Spec"=w1445) -> ("에러 출력"=w1446:errorcluster, "Data(str)"=w1447:string[][])  [unwired: 6 in, 1 out]
      }
      n392 = Index Array(array=w1440) -> (element=w1439:string[][])  [unwired: 3 in]
    }
    frame "Mass_1_1", "Mass_1_2", "Mass_1_3" {
      n393 = Unbundle By Name(w1475) -> ("분해능"=w1474:string, "문자열 1"=w1464:string)
      n394 = Index Array(array=w1489) -> (element=w1488:refnum<vi>)  [unwired: 1 in]
      n395 = Array Subset(array=w1469, index (col)=0 ("인덱스"), length (col)=2 ("길이")) -> (w1457:string[][])  [unwired: 2 in]
      n396 = Search/Split String(string=w1474, search string/char (-)="." ("검색 문자열/문자 (-)")) -> (match + rest of string=w1472:string)  [unwired: 1 in, 2 out]
      n397 = property class="Tbl (엄격한)"(reference=w1488, error in=w1461) -> (reference out=w1478:refnum<vi>, error out=w1476:errorcluster, "Value"=w1481:string[][])
      n398 = String Length(string=w1472) -> (length=w1471:i32)
      n399 = Decrement(x=w1471) -> (x-1=w1470:i32)
      n400 = Fract/Exp String To Number(string=w1481) -> (number=w1485:dbl[][])  [unwired: 3 in, 1 out]
      n401 = Index Array(array=w1485) -> (element=w1482:dbl[])  [unwired: 2 in]
      n402 = Index Array(array=w1482) -> (element=w1483:dbl)  [unwired: 1 in]
      n403 = Subtract(x=w1482, y=w1483) -> (x-y=w1484:dbl[])
      n404 = for {
        tunnel: w1484 -> [w1497] mode=indexing
        tunnel: [w1496] -> w1479 mode=indexing
        tunnel: w1470 -> [w1495]
        n405 = Number To Fractional String(number=w1497, precision (6)=w1495) -> (F-format string=w1496:string)  [unwired: 2 in]
      }
      n406 = Index Array(array=w1481) -> (element=w1480:string[])  [unwired: 2 in]
      n407 = Build Array(w1464) -> (w1463:string[])
      n408 = Build Array(w1480, w1479) -> (w1465:string[][])
      n409 = property class="Tbl (엄격한)"(reference=w1478, error in=w1476, "Value"=w1465) -> (error out=w1477:errorcluster)  [unwired: 1 out]
      n410 = Insert Into Array(array=w1465, new element=w1463) -> (w1466:string[][])  [unwired: 2 in]
      n411 = call "Variables Data IO.vi"("Write blank data ?(F)"=TRUE ("Clear data ?"), "Select"=Cmd_Var_Data_IO."Result2", "error in"=w1477, "Data In"=w1466, "Func_ext"=w1462) -> ("error out"=w1459:errorcluster)  [unwired: 4 in, 2 out]
      n412 = for {
        tunnel: w1454 -> [w1494] mode=indexing
        tunnel: [w1493] -> w1460 mode=indexing
        tunnel: w1457 -> [w1490]
        shift-right: [w1491] -> w1458
        shift-left: w1459 -> [w1492]
        n413 = call "Cell color by inspection (2D).vi"("에러 입력(에러 없음)"=w1492, "테이블 입력"=w1494, "Spec"=w1490) -> ("에러 출력"=w1491:errorcluster, "Data(str)"=w1493:string[][])  [unwired: 6 in, 1 out]
      }
      n414 = Index Array(array=w1460) -> (element #1=w1456:string[][], element #2=w1455:string[][])  [unwired: 6 in]
    }
    frame "Mass_2_1" {
      w1525 = 1 ("인덱스 (행)")
      n415 = Index Array(array=w1542) -> (element=w1541:refnum<vi>)  [unwired: 1 in]
      n416 = Unbundle By Name(w1516) -> ("숫자형 1"=w1510:i32, "숫자형 2"=w1509:i32, "문자열 1"=w1512:string, "숫자형 1"=w1499:i32, "문자배열 2D"=w1513:string[][])
      n417 = Index Array(array=w1505) -> (element #1=w1504:refnum<vi>, element #2=w1503:refnum<vi>, element #3=w1502:refnum<vi>)  [unwired: 3 in]
      n418 = Unbundle By Name(w1516) -> ("숫자형 1"=w1511:i32)
      n419 = property class="Tbl (엄격한)"(reference=w1541) -> (reference out=w1539:refnum<vi>, "DisabledEnum"=w1498:T4, "Value"=w1521:string[][])  [unwired: 1 in, 1 out]
      n420 = Build Array(w1503, w1502) -> (w1501:refnum<vi>[])
      n421 = Index Array(array=w1513, index (row)=w1499, index (col)=0 ("비활성화된 인덱스 (열)")) -> (element=w1531:string)
      n422 = Search/Split String(string=w1531, search string/char (-)="." ("검색 문자열/문자 (-)")) -> (match + rest of string=w1530:string)  [unwired: 1 in, 2 out]
      n423 = String Length(string=w1530) -> (length=w1519:i32)
      n424 = Equal To 0?(x=w1519) -> (x = 0?=w1520:bool)
      n425 = Decrement(x=w1519) -> (x-1=w1518:i32)
      n426 = Select(t=w1519, s=w1520, f=w1518) -> (s? t:f=w1517:i32)
      n427 = for {
        tunnel: [w1562] -> w1508 mode=indexing
        tunnel: w1517 -> [w1566]
        tunnel: w1501 -> [w1565] mode=indexing
        n428 = property class="Tbl (엄격한)"(reference=w1565) -> (reference out=w1563:refnum<vi>, "Value"=w1564:string[][])  [unwired: 1 in, 1 out]
        n429 = for {
          tunnel: w1564 -> [w1569] mode=indexing
          tunnel: [w1568] -> w1562 mode=indexing
          tunnel: w1566 -> [w1567]
          n430 = for {
            tunnel: w1569 -> [w1570] mode=indexing
            tunnel: [w1572] -> w1568 mode=indexing
            tunnel: w1567 -> [w1571]
            n431 = case shown="기본" w1570 {
              selector: w1570 -> [w1573 w1574]
              tunnel: [w1573 w1576] -> w1572
              tunnel: w1571 -> [_ w1575]
              frame "" {
              }
              frame Default {
                n432 = Fract/Exp String To Number(string=w1574) -> (number=w1577:dbl)  [unwired: 3 in, 1 out]
                n433 = Number To Fractional String(number=w1577, precision (6)=w1575) -> (F-format string=w1576:string)  [unwired: 2 in]
              }
            }
          }
        }
        n434 = property class="Tbl (엄격한)"(reference=w1563, "Value"=w1562) -> ()  [unwired: 1 in, 2 out]
      }
      n435 = Index Array(array=w1508) -> (element #1=w1507:string[][], element #2=w1506:string[][])  [unwired: 6 in]
      n436 = call "Calcu_Weight.vi"("Measured"=w1507, "공기밀도"=w1512, "측정횟수"=w1509, "분해능자리수"=w1517, "분동식별표기"=w1521) -> ("X=S-T"=w1527:string[][], "분동식별표기"=w1500:string[][])  [unwired: 5 in]
      n437 = property class="Tbl (엄격한)"(reference=w1504) -> ("Value"=w1523:string[][])  [unwired: 1 in, 2 out]
      n438 = case shown="\"Enabled\"" w1498 {
        tunnel: w1540 -> [w1561 _]
        tunnel: w1539 -> [w1549 _]
        tunnel: w1510 -> [w1545 _]
        tunnel: w1500 -> [w1544 _]
        frame "Enabled" {
          w1547 = 1 ("인덱스 (행)")
          n439 = Index Array(array=w1561, index (row) #1=w1545, index (col) #1=0 ("비활성화된 인덱스 (열)")) -> (element #1=w1543:string, element #2=w1556:string, element #3=w1557:string)  [unwired: 4 in]
          n440 = Bundle("인덱스 (행)"=w1547, "인덱스 (행)"=w1547) -> (w1548:cluster{"인덱스 (행)":i32, "인덱스 (행)":i32})  [unwired: 1 in]
          n441 = Index Array(array=w1544, index (row)=w1547, index (col)=w1547) -> (element=w1560:string)
          n442 = Fract/Exp String To Number(string=w1556) -> (number=w1555:dbl)  [unwired: 3 in, 1 out]
          n443 = call "Unit Conversion.vi"("환산단위"=w1557, "입력단위"="g", "입력값"=w1560) -> ("환산값 (DBL)"=w1553:dbl)  [unwired: 3 in, 5 out]
          n444 = Fract/Exp String To Number(string=w1543) -> (number=w1554:dbl)  [unwired: 3 in, 1 out]
          n445 = In Range and Coerce(upper limit=w1555, x=w1553, lower limit=w1554) -> (In Range?=w1550:bool)  [unwired: 1 out]
          n446 = Select(t=u32 16448250, s=w1550, f=u32 16711680) -> (s? t:f=w1546:u32)
          n447 = property class="Tbl (엄격한)"(reference=w1549, "Active Cell"=w1548, "Cell BG Color"=w1546, "Value"=w1544) -> ()  [unwired: 1 in, 2 out]
        }
        frame Default {
        }
      }
      n448 = Replace Array Subset(array=w1523, new element #1=w1507, index (row) #1=w1525, index (col) #1=0 ("비활성화된 인덱스 (열)"), new element #2=w1506, index (row) #2=w1525, index (col) #2=2 ("비활성화된 인덱스 (행)")) -> (w1522:string[][])
      n449 = call "Variables Data IO.vi"("Select"=Cmd_Var_Data_IO."Result", "error in"=w1514, "Func_ext"=w1515) -> ("error out"=w1534:errorcluster, "Data Out"=w1537:string[][])  [unwired: 6 in, 1 out]
      n450 = Multiply(x=3 ("길이"), y=w1511) -> (x*y=w1536:i32)
      n451 = Replace Array Subset(array=w1537, new element=w1522, index (row)=0 ("비활성화된 인덱스 (행)"), index (col)=w1536) -> (w1532:string[][])
    }
    frame "Mass_2_2" {
      w1600 = 1 ("인덱스 (행)")
      n452 = Index Array(array=w1623) -> (element=w1622:refnum<vi>)  [unwired: 1 in]
      n453 = Unbundle By Name(w1582) -> ("문자열 1"=w1579:string, "숫자형 1"=w1581:i32, "문자배열 2D"=w1583:string[][])
      n454 = property class="Tbl (엄격한)"(reference=w1622) -> (reference out=w1620:refnum<vi>, "DisabledEnum"=w1578:T4, "Value"=w1592:string[][])  [unwired: 1 in, 1 out]
      n455 = Unbundle By Name(w1582) -> ("숫자형 1"=w1580:i32)
      n456 = Index Array(array=w1612) -> (element #1=w1595:refnum<vi>, element #2=w1594:refnum<vi>, element #3=w1604:refnum<vi>)  [unwired: 3 in]
      n457 = Index Array(array=w1583, index (row)=w1581, index (col)=0 ("비활성화된 인덱스 (열)")) -> (element=w1611:string)
      n458 = property class="Tbl (엄격한)"(reference=w1594) -> (reference out=w1605:refnum<vi>, "Value"=w1607:string[][])  [unwired: 1 in, 1 out]
      n459 = property class="Tbl (엄격한)"(reference=w1604) -> (reference out=w1602:refnum<vi>, "Value"=w1603:string[][])  [unwired: 1 in, 1 out]
      n460 = Search/Split String(string=w1611, search string/char (-)="." ("검색 문자열/문자 (-)")) -> (match + rest of string=w1610:string)  [unwired: 1 in, 2 out]
      n461 = String Length(string=w1610) -> (length=w1589:i32)
      n462 = Equal To 0?(x=w1589) -> (x = 0?=w1590:bool)
      n463 = Decrement(x=w1589) -> (x-1=w1588:i32)
      n464 = Select(t=w1589, s=w1590, f=w1588) -> (s? t:f=w1587:i32)
      n465 = for {
        tunnel: w1607 -> [w1656] mode=indexing
        tunnel: [w1655] -> w1593 mode=indexing
        tunnel: w1587 -> [w1654]
        n466 = for {
          tunnel: w1656 -> [w1657] mode=indexing
          tunnel: [w1659] -> w1655 mode=indexing
          tunnel: w1654 -> [w1658]
          n467 = case shown="기본" w1657 {
            selector: w1657 -> [w1660 w1661]
            tunnel: [w1660 w1663] -> w1659
            tunnel: w1658 -> [_ w1662]
            frame "" {
            }
            frame Default {
              n468 = Fract/Exp String To Number(string=w1661) -> (number=w1664:dbl)  [unwired: 3 in, 1 out]
              n469 = Number To Fractional String(number=w1664, precision (6)=w1662) -> (F-format string=w1663:string)  [unwired: 2 in]
            }
          }
        }
      }
      n470 = for {
        tunnel: w1603 -> [w1645] mode=indexing
        tunnel: [w1644] -> w1597 mode=indexing
        tunnel: w1587 -> [w1643]
        n471 = for {
          tunnel: w1645 -> [w1646] mode=indexing
          tunnel: [w1648] -> w1644 mode=indexing
          tunnel: w1643 -> [w1647]
          n472 = case shown="기본" w1646 {
            selector: w1646 -> [w1649 w1650]
            tunnel: [w1649 w1652] -> w1648
            tunnel: w1647 -> [_ w1651]
            frame "" {
            }
            frame Default {
              n473 = Fract/Exp String To Number(string=w1650) -> (number=w1653:dbl)  [unwired: 3 in, 1 out]
              n474 = Number To Fractional String(number=w1653, precision (6)=w1651) -> (F-format string=w1652:string)  [unwired: 2 in]
            }
          }
        }
      }
      n475 = call "Calcu_Weight.vi"("Measured"=w1593, "공기밀도"=w1579, "측정횟수"=5, "분해능자리수"=w1587, "분동식별표기"=w1592) -> ("X=S-T"=w1606:string[][], "분동식별표기"=w1591:string[][])  [unwired: 5 in]
      n476 = case shown="\"Enabled\"" w1578 {
        tunnel: w1621 -> [w1642 _]
        tunnel: w1620 -> [w1629 _]
        tunnel: w1591 -> [w1625 _]
        tunnel: w1581 -> [w1624 _]
        frame "Enabled" {
          w1627 = 1 ("인덱스 (행)")
          n477 = Index Array(array=w1642, index (row) #1=w1624, index (col) #1=0 ("비활성화된 인덱스 (열)")) -> (element #1=w1635:string, element #2=w1637:string, element #3=w1638:string)  [unwired: 4 in]
          n478 = Fract/Exp String To Number(string=w1635) -> (number=w1634:dbl)  [unwired: 3 in, 1 out]
          n479 = Index Array(array=w1625, index (row)=w1627, index (col)=w1627) -> (element=w1641:string)
          n480 = Fract/Exp String To Number(string=w1637) -> (number=w1636:dbl)  [unwired: 3 in, 1 out]
          n481 = call "Unit Conversion.vi"("환산단위"=w1638, "입력단위"="g", "입력값"=w1641) -> ("환산값 (DBL)"=w1633:dbl)  [unwired: 3 in, 5 out]
          n482 = In Range and Coerce(upper limit=w1636, x=w1633, lower limit=w1634) -> (In Range?=w1630:bool)  [unwired: 1 out]
          n483 = Select(t=u32 16448250, s=w1630, f=u32 16711680) -> (s? t:f=w1626:u32)
          n484 = Bundle("인덱스 (행)"=w1627, "인덱스 (행)"=w1627) -> (w1628:cluster{"인덱스 (행)":i32, "인덱스 (행)":i32})  [unwired: 1 in]
          n485 = property class="Tbl (엄격한)"(reference=w1629, "Active Cell"=w1628, "Cell BG Color"=w1626, "Value"=w1625) -> ()  [unwired: 1 in, 2 out]
        }
        frame Default {
        }
      }
      n486 = property class="Tbl (엄격한)"(reference=w1602, "Value"=w1597) -> ()  [unwired: 1 in, 2 out]
      n487 = property class="Tbl (엄격한)"(reference=w1595) -> ("Value"=w1598:string[][])  [unwired: 1 in, 2 out]
      n488 = property class="Tbl (엄격한)"(reference=w1605, "Value"=w1593) -> ()  [unwired: 1 in, 2 out]
      n489 = Replace Array Subset(array=w1598, new element #1=w1593, index (row) #1=w1600, index (col) #1=0 ("비활성화된 인덱스 (열)"), new element #2=w1597, index (row) #2=w1600, index (col) #2=2 ("비활성화된 인덱스 (행)")) -> (w1596:string[][])
      n490 = Multiply(x=3 ("길이"), y=w1580) -> (x*y=w1617:i32)
      n491 = call "Variables Data IO.vi"("Select"=Cmd_Var_Data_IO."Result", "error in"=w1585, "Func_ext"=w1584) -> ("error out"=w1615:errorcluster, "Data Out"=w1618:string[][])  [unwired: 6 in, 1 out]
      n492 = Replace Array Subset(array=w1618, new element=w1596, index (row)=0 ("비활성화된 인덱스 (행)"), index (col)=w1617) -> (w1613:string[][])
    }
    frame "Pressure_3" {
      n493 = Unbundle By Name(w1677) -> ("문자배열 1D"=w1674:string[])
      n494 = Build Array(w1674) -> (w1672:string[][])
      n495 = Array Subset(array=w1678, index (col)=0 ("인덱스"), length (col)=2 ("길이")) -> (w1671:string[][])  [unwired: 2 in]
      n496 = call "Variables Data IO.vi"("Select"=Cmd_Var_Data_IO."Result2", "error in"=w1673, "Data In"=w1672, "Func_ext"=w1675) -> ("error out"=w1669:errorcluster)  [unwired: 5 in, 2 out]
      n497 = for {
        tunnel: w1671 -> [w1685]
        tunnel: w1670 -> [w1684] mode=indexing
        tunnel: [w1682] -> w1668 mode=indexing
        shift-right: [w1681] -> w1667
        shift-left: w1669 -> [w1683]
        n498 = call "Cell color by inspection (2D).vi"("에러 입력(에러 없음)"=w1683, "테이블 입력"=w1684, "Spec"=w1685) -> ("에러 출력"=w1681:errorcluster, "Data(str)"=w1682:string[][])  [unwired: 6 in, 1 out]
      }
      n499 = Index Array(array=w1668) -> (element #1=w1666:string[][], element #2=w1665:string[][])  [unwired: 6 in]
    }
    frame "Pressure_4" {
      n500 = Unbundle By Name(w1692) -> ("문자배열 1D"=w1687:string[])
      n501 = Build Array(w1687) -> (w1686:string[][])
      n502 = call "Variables Data IO.vi"("Select"=Cmd_Var_Data_IO."Result2", "error in"=w1691, "Data In"=w1686, "Func_ext"=w1690) -> ("error out"=w1688:errorcluster)  [unwired: 5 in, 2 out]
      n503 = Array Subset(array=w1699, index (col)=0 ("인덱스"), length (col)=2 ("길이")) -> (w1698:string[][])  [unwired: 2 in]
      n504 = for {
        tunnel: w1698 -> [w1706]
        tunnel: w1697 -> [w1705] mode=indexing
        tunnel: [w1703] -> w1696 mode=indexing
        shift-right: [w1702] -> w1695
        shift-left: w1688 -> [w1704]
        n505 = call "Cell color by inspection (2D).vi"("에러 입력(에러 없음)"=w1704, "테이블 입력"=w1705, "Spec"=w1706) -> ("에러 출력"=w1702:errorcluster, "Data(str)"=w1703:string[][])  [unwired: 6 in, 1 out]
      }
      n506 = Index Array(array=w1696) -> (element #1=w1694:string[][], element #2=w1693:string[][])  [unwired: 6 in]
    }
    frame Default {
      w1711 = TRUE ("Write blank data ?")
      # "INS_1=MEAS1, INS_2=MEAS2, INS_3=MEAS3"
      n507 = for {
        tunnel: w1721 -> [w1724] mode=indexing
        tunnel: [w1727] -> w1718 mode=indexing
        tunnel: w1720 -> [w1726]
        shift-right: [w1722] -> w1715
        shift-left: w1719 -> [w1723]
        n508 = Array Subset(array=w1726, index (col)=0 ("인덱스"), length (col)=2 ("길이")) -> (w1725:string[][])  [unwired: 2 in]
        n509 = call "Cell color by inspection (2D).vi"("에러 입력(에러 없음)"=w1723, "테이블 입력"=w1724, "Spec"=w1725) -> ("에러 출력"=w1722:errorcluster, "Data(str)"=w1727:string[][])  [unwired: 6 in, 1 out]
      }
      n510 = Index Array(array=w1718) -> (element #1=w1717:string[][], element #2=w1713:string[][], element #3=w1707:string[][])  [unwired: 9 in]
      n511 = call "Variables Data IO.vi"("Write blank data ?(F)"=w1711, "Select"=Cmd_Var_Data_IO."Result2", "error in"=w1715, "Data In"=w1713, "Func_ext"=w1714) -> ("error out"=w1710:errorcluster, "Func_ext Out"=w1708:string)  [unwired: 4 in, 1 out]
      n512 = call "Variables Data IO.vi"("Write blank data ?(F)"=w1711, "Select"=Cmd_Var_Data_IO."Result3", "error in"=w1710, "Data In"=w1707, "Func_ext"=w1708) -> ("error out"=w1709:errorcluster)  [unwired: 4 in, 2 out]
    }
  }
  "Data (spec 적용)" <- w21
  "Data (spec 미적용)" <- w20
  "Data 3D" <- w2
  "spec DBL" <- w1
  n513 = call "Variables Data IO.vi"("Write blank data ?(F)"=TRUE ("Write blank data ?"), "Select"=Cmd_Var_Data_IO."Result", "error in"=w24, "Data In"=w21, "Func_ext"="Func ext") -> ("error out"=w8:errorcluster, "Func_ext Out"=w6:string)  [unwired: 4 in, 1 out]
  n514 = call "Variables Data IO.vi"("Write blank data ?(F)"=FALSE ("Write blank data ?(T)"), "Select"=Cmd_Var_Data_IO."Result_ADJ", "error in"=w8, "Data In"=w4, "Func_ext"=w6) -> ("error out"=→"error out":errorcluster)  [unwired: 4 in, 2 out]
